vi "FRF_Koherenz_THD_Single_Shot.vi"(6 "error in":errorcluster, 7 "Peiker_Stepped Sweep Settings":T1={"Input Settings"={"IEPE min time to settle [s]"=0.0, "Responce Channel Settings"={"DSA response channel settings"={"coupling"=10045, "enable IEPE excitation"=FALSE, "IEPE current [mA]"=4.0}, "response channel info"={"sensor sensitivity"=200.0, "engineering units"=2, "dB reference"=2e-05, "custom label"="EU", "weighting filter"=0, "pregain"=0.0}, "AI response settings"={"response channel"="SOUNDACQ/ai1", "max value [V]"=10.0, "min value [V]"=-10.0, "terminal configuration"=-1}}, "Stimulus Channel Settings"={"AI stimulus settings"={"stimulus channel"="SOUNDACQ/ai0", "max value [V]"=10.0, "min value [V]"=-10.0, "terminal configuration"=-1}, "DSA stimulus channel settings"={"coupling"=10045, "enable IEPE excitation"=TRUE, "IEPE current [mA]"=4.0}, "stimulus channel info"={"sensor sensitivity"=11.4, "engineering units"=2, "dB reference"=2e-05, "custom label"="EU", "weighting filter"=0, "pregain"=0.0}}}, "Output Settings"={"AO source settings"={"excitation channel"="SOUNDACQ/ao0", "max value [V]"=10.0, "min value [V]"=-10.0, "terminal configuration"=-1}}} {"Output Settings"."AO source settings"."terminal configuration" items=["Default"=-1, "RSE"=10083, "Differential"=10106, "Pseudodifferential"=12529]; "Output Settings"."AO source settings"."min value [V]" format="%0.2f"; "Output Settings"."AO source settings"."max value [V]" format="%0.2f"; "Input Settings"."Stimulus Channel Settings"."stimulus channel info"."pregain" format="%.2f"; "Input Settings"."Stimulus Channel Settings"."stimulus channel info"."weighting filter" items=["Linear", "A-weighting", "B-weighting", "C-weighting", "ITU-R 468-4", "Dolby", "CCITT", "C-message", "Wb", "Wc", "Wd", "We", "Wf", "Wh", "Wj", "Wk", "Wm", "AES17 20 kHz lowpass", "AES17 40 kHz lowpass", "AES17 20 kHz highpass", "AES17 40 kHz highpass"]; "Input Settings"."Stimulus Channel Settings"."stimulus channel info"."dB reference" format="%^.1e"; "Input Settings"."Stimulus Channel Settings"."stimulus channel info"."engineering units" items=["custom..."=0, "V"=1, "A"=21, "C"=30, "pC"=31, "s"=32, "-"=29, "Pa"=2, "N"=20, "g"=3, "m/s^2"=4, "m/s"=5, "m"=6, "mm/s"=12, "mm"=13, "micron/s"=14, "micron"=15, "in/s^2"=7, "in/s"=8, "in"=9, "mil/s"=10, "mil"=11, "rad/s^2"=16, "rad/s"=17, "rad"=18, "deg/s^2"=26, "deg/s"=27, "deg"=28, "RPM"=22, "cycle/s^2"=23, "Hz"=24, "cycle"=25, "strain"=19]; "Input Settings"."Stimulus Channel Settings"."stimulus channel info"."sensor sensitivity" format="%#_5f"; "Input Settings"."Stimulus Channel Settings"."DSA stimulus channel settings"."IEPE current [mA]" format="%.1f"; "Input Settings"."Stimulus Channel Settings"."DSA stimulus channel settings"."coupling" items=["AC"=10045, "DC"=10050, "GND"=10066]; "Input Settings"."Stimulus Channel Settings"."AI stimulus settings"."terminal configuration" items=["Default"=-1, "RSE"=10083, "NRSE"=10078, "Differential"=10106, "Pseudodifferential"=12529]; "Input Settings"."Stimulus Channel Settings"."AI stimulus settings"."min value [V]" format="%.2f"; "Input Settings"."Stimulus Channel Settings"."AI stimulus settings"."max value [V]" format="%.2f"; "Input Settings"."Responce Channel Settings"."AI response settings"."terminal configuration" items=["Default"=-1, "RSE"=10083, "NRSE"=10078, "Differential"=10106, "Pseudodifferential"=12529]; "Input Settings"."Responce Channel Settings"."AI response settings"."min value [V]" format="%.2f"; "Input Settings"."Responce Channel Settings"."AI response settings"."max value [V]" format="%.2f"; "Input Settings"."Responce Channel Settings"."response channel info"."pregain" format="%.2f"; "Input Settings"."Responce Channel Settings"."response channel info"."weighting filter" items=["Linear", "A-weighting", "B-weighting", "C-weighting", "ITU-R 468-4", "Dolby", "CCITT", "C-message", "Wb", "Wc", "Wd", "We", "Wf", "Wh", "Wj", "Wk", "Wm", "AES17 20 kHz lowpass", "AES17 40 kHz lowpass", "AES17 20 kHz highpass", "AES17 40 kHz highpass"]; "Input Settings"."Responce Channel Settings"."response channel info"."dB reference" format="%^.1e"; "Input Settings"."Responce Channel Settings"."response channel info"."engineering units" items=["custom..."=0, "V"=1, "A"=21, "C"=30, "pC"=31, "s"=32, "-"=29, "Pa"=2, "N"=20, "g"=3, "m/s^2"=4, "m/s"=5, "m"=6, "mm/s"=12, "mm"=13, "micron/s"=14, "micron"=15, "in/s^2"=7, "in/s"=8, "in"=9, "mil/s"=10, "mil"=11, "rad/s^2"=16, "rad/s"=17, "rad"=18, "deg/s^2"=26, "deg/s"=27, "deg"=28, "RPM"=22, "cycle/s^2"=23, "Hz"=24, "cycle"=25, "strain"=19]; "Input Settings"."Responce Channel Settings"."response channel info"."sensor sensitivity" format="%#_5f"; "Input Settings"."Responce Channel Settings"."DSA response channel settings"."IEPE current [mA]" format="%.1f"; "Input Settings"."Responce Channel Settings"."DSA response channel settings"."coupling" items=["AC"=10045, "DC"=10050, "GND"=10066]; "Input Settings"."IEPE min time to settle [s]" format="%.1f"}, 8 "timeout(s)":dbl=10.0, 9 "Std_Deviation_Thresold":dbl=0.04, 10 "Excitation_amplitude(Vpeak)":dbl=0.35 min=0.0 format="%.3f", 11 "dB SPL":dbl=94.0502) -> (0 "mean":dbl=0.5389452537133329, 3 "Sensitivity(mVeff/Pa)":dbl=314.40385852797573, 4 "error out":errorcluster)   [LabVIEW 2018]
uses:
  <vilib>/addons/_NISVFA/_Shared subVIs/Controls/svc_Window [Dual FFT].ctl
  Peiker_Stepped Sweep Settings.ctl
  <vilib>/addons/_NISVFA/_Shared subVIs/Controls/svc_DSA Channel Settings.ctl
  <vilib>/addons/_NISVFA/_Shared subVIs/Controls/svc_Channel Info.ctl
  <vilib>/addons/_NISVFA/_Shared subVIs/Controls/svc_Engineering Units Text Ring.ctl
  <vilib>/addons/_NISVFA/_Shared subVIs/Controls/svc_Weighting Filter Text Ring.ctl
  <vilib>/DAQmx/write.llb/DAQmx Write (Analog 1D DBL 1Chan NSamp).vi
  <vilib>/DAQmx/read.llb/DAQmx Read (Analog 1D Wfm NChan NSamp).vi
  THD_Mess_Status.vi
  <vilib>/DAQmx/create/channels.llb/DAQmx Create Channel (AI-Voltage-Basic).vi
  <vilib>/DAQmx/configure/timing.llb/DAQmx Timing (Sample Clock).vi
  <vilib>/DAQmx/create/channels.llb/DAQmx Create Channel (AO-Voltage-Basic).vi
  <vilib>/DAQmx/configure/trigger.llb/DAQmx Start Trigger (Digital Edge).vi
  <vilib>/DAQmx/miscellaneous.llb/DAQmx Fill In Error Info.vi
  <vilib>/addons/_NISVFA/_Baseband FFT/SVFA Frequency Response (1x1) (Mag-Phase).vi
  <vilib>/addons/Sound and Vibration/svt_Distortion/SVT THD and Harmonic Components (Time) (1 Ch).vi
  <vilib>/addons/_NISVFA/_Baseband FFT/SVFA Power Spectrum (1 Ch).vi
  <vilib>/Analysis/NI_AALBase.lvlib
  <vilib>/addons/Sound and Vibration/svt_Distortion/SoundVib_Distortion.lvlib
  <resource>/objmgr/daqmx.rc
panel:
  out "Array 4":dbl[](array[numeric])
  out "Array 3":dbl[](array[numeric])
  out "Array 2":dbl[](array[numeric])
  out "standard deviation":dbl=0.020322606714807942
  out "Array":u32[](array[numeric])=[21, 20, 29, 17, 19, 19, 19, 19, 25, 19, 20, 18, 18, 22, 20, 18, 22, 19, 19, 23, 19, 19, 21, 20, 20, 19, 20, 19]
  out "XY Graph 3":cluster{dbl[], dbl[]}[](graph)=[{[0.021, 0.041, 0.07, 0.08700000000000001, 0.10600000000000001, 0.125, 0.144, 0.16299999999999998, 0.18799999999999997, 0.20699999999999996, 0.22699999999999995, 0.24499999999999994, 0.26299999999999996, 0.285, 0.305, 0.323, 0.34500000000000003, 0.36400000000000005, 0.38300000000000006, 0.4060000000000001, 0.4250000000000001, 0.4440000000000001, 0.46500000000000014, 0.48500000000000015, 0.5050000000000001, 0.5240000000000001, 0.5440000000000002, 0.5630000000000002], [0.5, 0.5, 0.5, 0.5, 0.5, 0.5, 0.5, 0.5, 0.5, 0.5, 0.5, 0.5, 0.5, 0.5, 0.5, 0.5, 0.5, 0.5, 0.5, 0.5, 0.5, 0.5, 0.5, 0.5, 0.5, 0.5, 0.5, 0.5389452537133329]}, {[0.021, 0.041, 0.07, 0.08700000000000001, 0.10600000000000001, 0.125, 0.144, 0.16299999999999998, 0.18799999999999997, 0.20699999999999996, 0.22699999999999995, 0.24499999999999994, 0.26299999999999996, 0.285, 0.305, 0.323, 0.34500000000000003, 0.36400000000000005, 0.38300000000000006, 0.4060000000000001, 0.4250000000000001, 0.4440000000000001, 0.46500000000000014, 0.48500000000000015, 0.5050000000000001, 0.5240000000000001, 0.5440000000000002, 0.5630000000000002], [0.5, 0.5, 0.5, 0.5, 0.5, 0.5, 0.5, 0.5, 0.5, 0.5, 0.5, 0.5, 0.5, 0.5, 0.5, 0.5, 0.5, 0.5, 0.5, 0.5, 0.5, 0.5, 0.5, 0.5, 0.5, 0.5, 0.5, 0.020322606714807942]}]
  in  "Coh Faktor Thresold":dbl=999.98 format="%#_10g"
  out "XY Graph 2":cluster{dbl[], dbl[]}(graph)={[0.021, 0.041, 0.07, 0.08700000000000001, 0.10600000000000001, 0.125, 0.144, 0.16299999999999998, 0.18799999999999997, 0.20699999999999996, 0.22699999999999995, 0.24499999999999994, 0.26299999999999996, 0.285, 0.305, 0.323, 0.34500000000000003, 0.36400000000000005, 0.38300000000000006, 0.4060000000000001, 0.4250000000000001, 0.4440000000000001, 0.46500000000000014, 0.48500000000000015, 0.5050000000000001, 0.5240000000000001, 0.5440000000000002, 0.5630000000000002], [0.0, 0.0, 0.0, 0.0, 0.0, 0.0, 0.0, 0.0, 0.0, 0.0, 0.545398761909948, 0.5338370932650872, 0.551146395387674, 0.5719764653070627, 0.5375454545895423, 0.537446460172108, 0.5808316642168437, 0.5322047145448163, 0.542195941406813, 0.5587662684664381, 0.535636496263525, 0.5091814361274755, 0.530595639527823, 0.5291564969244456, 0.5460569136668927, 0.5432199651402557, 0.5429647634305357, 0.513659110796227]}
  out "Big Sound Disturbances detected":i32=1
  out "Sound Pressure (Pa)":dbl=1.0081844522429841
  in  "swept sine settings":enum32{"DAQ Settings", "FRF Settings"}(tab)=enum."FRF Settings"
  out "input channel (response)":tag="SOUNDACQ/ai1"
  in  "propagation delay [samples]":i32=133 min=1 step=1
  out "input channel (stimulus)":tag="SOUNDACQ/ai0"
  out "output physical channel":tag="SOUNDACQ/ao0"
  out "actual update rate":dbl=50000.00001018634 format="%.2f"
  in  "sampling rate [Hz]":dbl=50000.0 format="%.2f"
  out "averages completed":dbl=5665.0
  in  "restart averaging":bool
  in  "averaging parameters":T6={"averaging mode"=enum."RMS averaging", "weighting mode"=enum."Exponential", "number of averages"=2, "linear mode"=enum."One shot"} {"number of averages" min=1 step=1}
  in  "view":T7={"dB On"=TRUE, "unwrap phase"=FALSE, "convert to degree"=TRUE}
  in  "block size":i32=1000 min=128
  in  "window":T8=1 items=["None"=0, "Hanning"=1, "Hamming"=2, "Blackman-Harris"=3, "Exact Blackman"=4, "Blackman"=5, "Flat Top"=6, "4 Term B-Harris "=7, "7 Term B-Harris"=8, "Low Sidelobe"=9, "Force - Exponential"=10, "Blackman Nuttall"=11, "Triangle"=30, "Bartlett-Hanning"=31, "Bohman"=32, "Parzen"=33, "Welch"=34, "Kaiser"=60, "Dolph-Chebyshev"=61, "Gaussian"=62]
  in  "Tab Control":enum32{"Getting Started", "Time Record", "FRF"}(tab)=enum."FRF"
  in  "Getting Started Text":string="GETTING STARTED\n\nThis VI measures the Frequency Response Function (FRF) of a device under test (DUT).  It generates a broadband stimulus signal to excite the DUT.  The magnitude and phase of the DUT output are compared to the stimulus signal to calculate the FRF.  \n\nRefer to the wiring diagram to physically connect the DSA or DAQ device to the DUT.  This example uses two analog input channels and one analog output channel.  Note that the analog output is connected to both the DUT input and to the first analog input channel on the measurement device.  \n\nThe wiring diagram assumes that you use the default channel settings.  If you change the channel settings in the VI front panel you should adjust the physical connections appropriately.\n\nNI strongly recommends that you take precautions to limit the effects of out-of-band aliasing in your frequency domain measurements.  DSA devices use transparent digital and analog hardware filtering to eliminate aliased input and output frequencies.  Multifunction DAQ devices are more susceptible to the effects of aliased frequencies.  If you are using a non-DSA measurement device, we recommend addressing potential aliasing through high sampling rates, built-in analog filters on S Series devices, and/or external analog filters.\n\n\nKEY PARAMETERS\n\nDAQ Configuration:  device propagation delay [samples]\n\nThis parameter quantifies the time, measured in sample intervals, between when a sample of data is generated on analog output and when it is read on the analog input.  Common sources of delay are analog or digital filters and propagation time for acoustical or mechanical signals.  The combined delay of the digital anti-aliasing and anti-imaging filters on the NI PCI-4451 and PCI-4551 devices is approximately 77 samples.  When using a multifunction E Series or S Series device, we recommend entering a delay of 1 sample.  An easy way to determine this delay for any given measurement system is to run SVT Measure Propagation Delay.vi.  This VI is available from the LabVIEW Functions palette under Sound and Vibration >> Calibration.\n\n\nSource Settings:  signal type\n\nThis control allows you to specify the type of stimulus signal you would like to generate.  All of the available signal sources are broadband stimuli with frequency content ranging from just above DC to the value specified in the \"Maximum Frequency of Interest\" control.  Note that if you use the \"Chirp\" or \"Frequency flat chirp\" signal types, you should select \"None\" for the window type.\n\nSource Settings:  maximum frequency of interest [Hz]\n\nThis setting controls the sampling rate for input and output.  The sampling rate is 2.5 times the value of this control.  Reducing the maximum frequency of interest may help if you encounter issues of data transfer bandwidth.\n\nMeasurement Settings:  frequency resolution [Hz]\n\nThis setting controls the width of a single frequency bin in the frequency response measurement.  Improving the frequency resolution requires more data points per average. Thus, the acquisition block size increases with finer frequency resolutions.  Improving (i.e. reducing) the frequency resolution may help if you encounter issues of data transfer bandwidth. \n\nMeasurement Settings:  window\n\nThis setting controls the time-domain window applied to the input signals before the frequency response function is calculated.  If you use the \"Chirp\" or \"Frequency flat chirp\" excitation types, you should not apply a window.\n\n\nMeasurement Settings:  settle time [s]\n\nThis control allows you to specify a time interval between when the stimulus generation starts and when the measurement actually begins. This time interval will be coerced to an integer number of data blocks.  If your DUT has a significant transient response to the start of a stimulus signal, select the appropriate settle time to allow this transient response to pass.\n"
  out "time record 2":waveform(dbl)[](graph)=[{"t0"=timestamp(3568218948.523604 s since 1904-01-01), "dt"=1.9999999995925458e-05, "Y"=array[1000 elements], "attributes"=variant("NI_ChannelName"=variant(string "stimulus"), "NI_UnitDescription"=variant(string "Volts"))}, {"t0"=timestamp(3568218948.523604 s since 1904-01-01), "dt"=1.9999999995925458e-05, "Y"=array[1000 elements], "attributes"=variant("NI_ChannelName"=variant(string "response"), "NI_UnitDescription"=variant(string "Volts"))}]
  out "Waveform Graph":dbl[](graph)=[0.0, 0.04386663174750649, 0.08704146050769919, 0.1288435934396373, 0.16861378593560036, 0.20572483830236563, 0.23959148707504105, 0.26967963497152625, 0.2955147739257053, 0.31668946836310685, 0.33286978070330375, 0.34380053775504105, 0.349309354949895, 0.349309354949895, 0.343800537755041, 0.3328697807033037, 0.3166894683631068, 0.2955147739257052, 0.2696796349715262, 0.23959148707504094, 0.20572483830236554, 0.16861378593560022, 0.12884359343963722, 0.08704146050769904, 0.04386663174750641, -1.4434796673928885e-16, -0.043866631747506574, -0.08704146050769931, -0.1288435934396374, -0.16861378593560047, -0.20572483830236568, -0.23959148707504113, -0.2696796349715263, -0.29551477392570535, -0.3166894683631069, -0.3328697807033038, -0.3438005377550411, -0.34930935494989507, -0.34930935494989507, -0.343800537755041, -0.33286978070330375, -0.31668946836310674, -0.29551477392570524, -0.2696796349715261, -0.23959148707504097, -0.2057248383023654, -0.16861378593560022, -0.12884359343963706, -0.08704146050769901, -0.04386663174750623, 1.9968971138109581e-16, 0.043866631747506754, 0.0870414605076994, 0.12884359343963755, 0.16861378593560059, 0.20572483830236585, 0.23959148707504127, 0.2696796349715264, 0.29551477392570547, 0.31668946836310696, 0.3328697807033039, 0.3438005377550411, 0.3493093549498952, 0.349309354949895, 0.3438005377550411, 0.33286978070330364, 0.3166894683631068, 0.2955147739257051, 0.2696796349715261, 0.23959148707504077, 0.20572483830236538, 0.16861378593560003, 0.128843593439637, 0.08704146050769881, 0.04386663174750615, -3.7825103292588036e-16, -0.04386663174750685, -0.08704146050769955, -0.12884359343963767, -0.1686137859356007, -0.20572483830236596, -0.23959148707504133, -0.2696796349715265, -0.29551477392570547, -0.3166894683631071, -0.33286978070330386, -0.3438005377550412, -0.34930935494989507, -0.3493093549498951, -0.34380053775504094, -0.3328697807033037, -0.31668946836310663, -0.29551477392570513, -0.2696796349715259, -0.23959148707504077, -0.2057248383023652, -0.1686137859356, -0.12884359343963683, -0.08704146050769876, -0.043866631747506, 4.652785860585762e-16, 0.043866631747506976, 0.08704146050769966, 0.12884359343963775, 0.1686137859356008, 0.20572483830236601, 0.23959148707504146, 0.2696796349715266, 0.29551477392570563, 0.3166894683631071, 0.33286978070330403, 0.34380053775504116, 0.3493093549498952, 0.349309354949895, 0.34380053775504105, 0.3328697807033036, 0.3166894683631067, 0.29551477392570497, 0.26967963497152597, 0.2395914870750406, 0.2057248383023652, 0.1686137859355998, 0.1288435934396368, 0.08704146050769856, 0.043866631747505935, -6.422136043446325e-16, -0.04386663174750707, -0.08704146050769981, -0.12884359343963786, -0.16861378593560095, -0.20572483830236613, -0.23959148707504155, -0.2696796349715267, -0.2955147739257057, -0.3166894683631072, -0.33286978070330403, -0.34380053775504127, -0.3493093549498951, -0.3493093549498951, -0.34380053775504094, -0.33286978070330364, -0.3166894683631066, -0.295514773925705, -0.2696796349715258, -0.23959148707504063, -0.20572483830236502, -0.1686137859355998, -0.12884359343963658, -0.08704146050769855, -0.04386663174750571, 6.790900307362957e-16, 0.04386663174750728, 0.08704146050769987, 0.12884359343963805, 0.168613785935601, 0.2057248383023663, 0.2395914870750416, 0.2696796349715268, 0.29551477392570574, 0.31668946836310724, 0.3328697807033041, 0.34380053775504127, 0.34930935494989523, 0.34930935494989507, 0.34380053775504105, 0.33286978070330353, 0.31668946836310663, 0.29551477392570485, 0.26967963497152586, 0.23959148707504044, 0.20572483830236507, 0.16861378593559959, 0.1288435934396366, 0.08704146050769831, 0.04386663174750571, -9.118275795874653e-16, -0.04386663174750731, -0.08704146050770008, -0.1288435934396381, -0.1686137859356012, -0.20572483830236638, -0.23959148707504177, -0.2696796349715269, -0.29551477392570585, -0.31668946836310735, -0.33286978070330414, -0.3438005377550414, -0.3493093549498952, -0.3493093549498952, -0.34380053775504094, -0.33286978070330364, -0.31668946836310646, -0.29551477392570497, -0.26967963497152564, -0.23959148707504052, -0.20572483830236482, -0.16861378593559964, -0.12884359343963636, -0.08704146050769833, -0.04386663174750547, 9.369539649348169e-16, 0.04386663174750753, 0.08704146050770015, 0.1288435934396383, 0.16861378593560128, 0.20572483830236651, 0.23959148707504188, 0.26967963497152697, 0.29551477392570596, 0.31668946836310735, 0.33286978070330425, 0.3438005377550413, 0.3493093549498953, 0.34930935494989507, 0.34380053775504105, 0.3328697807033035, 0.3166894683631066, 0.29551477392570474, 0.26967963497152575, 0.23959148707504027, 0.2057248383023649, 0.1686137859355994, 0.12884359343963642, 0.08704146050769809, 0.04386663174750549, -1.1476483283666405e-15, -0.043866631747507545, -0.08704146050770031, -0.12884359343963833, -0.1686137859356014, -0.20572483830236657, -0.23959148707504194, -0.2696796349715271, -0.29551477392570596, -0.3166894683631075, -0.3328697807033042, -0.3438005377550415, -0.3493093549498952, -0.34930935494989523, -0.3438005377550409, -0.33286978070330364, -0.3166894683631064, -0.29551477392570485, -0.26967963497152553, -0.23959148707504035, -0.20572483830236465, -0.16861378593559945, -0.12884359343963617, -0.0870414605076981, -0.04386663174750526, 1.1742316103832695e-15, 0.04386663174750774, 0.08704146050770038, 0.1288435934396385, 0.1686137859356015, 0.20572483830236668, 0.23959148707504208, 0.26967963497152714, 0.29551477392570613, 0.31668946836310746, 0.33286978070330436, 0.3438005377550414, 0.34930935494989535, 0.34930935494989507, 0.34380053775504105, 0.3328697807033034, 0.3166894683631065, 0.29551477392570463, 0.26967963497152564, 0.2395914870750401, 0.20572483830236474, 0.1686137859355992, 0.12884359343963622, 0.08704146050769787, 0.04386663174750527, -1.3799860776667061e-15, -0.04386663174750778, -0.08704146050770055, -0.12884359343963858, -0.1686137859356016, -0.2057248383023668, -0.23959148707504213, -0.26967963497152725, -0.29551477392570613, -0.31668946836310763, -0.3328697807033043, -0.34380053775504155, -0.34930935494989523, -0.34930935494989523, -0.3438005377550409, -0.3328697807033036, -0.3166894683631063, -0.2955147739257048, -0.26967963497152536, -0.23959148707504024, -0.20572483830236446, -0.16861378593559928, -0.12884359343963595, -0.08704146050769791, -0.04386663174750502, 1.3828050033151684e-15, 0.04386663174750799, 0.08704146050770059, 0.12884359343963872, 0.1686137859356017, 0.20572483830236687, 0.23959148707504224, 0.2696796349715273, 0.29551477392570624, 0.31668946836310763, 0.3328697807033044, 0.3438005377550415, 0.3493093549498954, 0.3493093549498951, 0.34380053775504105, 0.3328697807033034, 0.31668946836310646, 0.2955147739257046, 0.26967963497152553, 0.23959148707504, 0.2057248383023646, 0.16861378593559903, 0.12884359343963606, 0.08704146050769766, 0.04386663174750509, -1.6200419911821529e-15, -0.04386663174750797, -0.0870414605077008, -0.12884359343963875, -0.16861378593560186, -0.20572483830236696, -0.23959148707504235, -0.2696796349715274, -0.2955147739257063, -0.31668946836310774, -0.3328697807033044, -0.3438005377550416, -0.34930935494989535, -0.34930935494989523, -0.34380053775504094, -0.33286978070330353, -0.3166894683631063, -0.2955147739257047, -0.2696796349715253, -0.2395914870750401, -0.20572483830236435, -0.16861378593559911, -0.12884359343963578, -0.08704146050769773, -0.04386663174750482, 1.5683323238181723e-15, 0.04386663174750821, 0.08704146050770077, 0.12884359343963897, 0.16861378593560186, 0.20572483830236712, 0.23959148707504238, 0.2696796349715275, 0.29551477392570635, 0.3166894683631078, 0.3328697807033045, 0.3438005377550416, 0.3493093549498954, 0.3493093549498952, 0.343800537755041, 0.3328697807033034, 0.31668946836310635, 0.2955147739257045, 0.26967963497152536, 0.23959148707503988, 0.2057248383023644, 0.16861378593559886, 0.12884359343963583, 0.08704146050769745, 0.04386663174750486, -1.851539483798542e-15, -0.043866631747508184, -0.08704146050770104, -0.12884359343963894, -0.1686137859356021, -0.2057248383023671, -0.23959148707504258, -0.26967963497152747, -0.2955147739257065, -0.31668946836310774, -0.3328697807033046, -0.34380053775504155, -0.3493093549498954, -0.3493093549498951, -0.34380053775504094, -0.3328697807033034, -0.31668946836310624, -0.2955147739257045, -0.2696796349715252, -0.2395914870750399, -0.20572483830236418, -0.16861378593559892, -0.12884359343963558, -0.08704146050769754, -0.04386663174750459, 1.7499632927638065e-15, 0.04386663174750846, 0.08704146050770092, 0.12884359343963922, 0.16861378593560197, 0.20572483830236735, 0.23959148707504244, 0.2696796349715277, 0.29551477392570635, 0.3166894683631079, 0.3328697807033045, 0.34380053775504166, 0.34930935494989535, 0.3493093549498952, 0.3438005377550409, 0.33286978070330336, 0.31668946836310624, 0.2955147739257044, 0.26967963497152525, 0.23959148707503974, 0.20572483830236427, 0.1686137859355987, 0.1288435934396357, 0.08704146050769727, 0.04386663174750472, -2.041200325084147e-15, -0.043866631747508315, -0.08704146050770123, -0.12884359343963905, -0.16861378593560228, -0.2057248383023672, -0.23959148707504271, -0.2696796349715276, -0.29551477392570663, -0.31668946836310785, -0.33286978070330464, -0.3438005377550416, -0.34930935494989546, -0.3493093549498951, -0.34380053775504094, -0.33286978070330336, -0.3166894683631062, -0.2955147739257044, -0.2696796349715251, -0.23959148707503977, -0.20572483830236402, -0.16861378593559875, -0.1288435934396354, -0.08704146050769736, -0.04386663174750438, 1.9355244945847005e-15, 0.04386663174750867, 0.0870414605077011, 0.12884359343963941, 0.16861378593560214, 0.20572483830236754, 0.23959148707504258, 0.26967963497152786, 0.29551477392570646, 0.316689468363108, 0.33286978070330453, 0.3438005377550417, 0.34930935494989535, 0.3493093549498952, 0.3438005377550408, 0.3328697807033033, 0.31668946836310613, 0.2955147739257043, 0.2696796349715251, 0.23959148707503958, 0.20572483830236407, 0.1686137859355985, 0.12884359343963547, 0.08704146050769705, 0.0438666317475045, -2.2727655803363167e-15, -0.043866631747508524, -0.08704146050770145, -0.12884359343963925, -0.16861378593560247, -0.20572483830236735, -0.23959148707504288, -0.26967963497152764, -0.29551477392570674, -0.31668946836310785, -0.33286978070330475, -0.3438005377550416, -0.3493093549498955, -0.34930935494989507, -0.34380053775504094, -0.33286978070330325, -0.31668946836310613, -0.2955147739257043, -0.269679634971525, -0.23959148707503963, -0.20572483830236388, -0.1686137859355986, -0.1288435934396352, -0.08704146050769718, -0.04386663174750416, 2.119012159750716e-15, 0.043866631747508905, 0.08704146050770128, 0.12884359343963964, 0.1686137859356023, 0.20572483830236774, 0.23959148707504271, 0.269679634971528, 0.2955147739257066, 0.3166894683631082, 0.3328697807033046, 0.3438005377550418, 0.34930935494989535, 0.34930935494989523, 0.34380053775504077, 0.3328697807033033, 0.316689468363106, 0.29551477392570424, 0.2696796349715249, 0.23959148707503947, 0.20572483830236388, 0.16861378593559834, 0.12884359343963528, 0.08704146050769684, 0.043866631747504305, -2.5055505630325325e-15, -0.04386663174750871, -0.0870414605077017, -0.12884359343963941, -0.16861378593560272, -0.20572483830236749, -0.23959148707504313, -0.26967963497152775, -0.29551477392570696, -0.3166894683631079, -0.3328697807033049, -0.3438005377550416, -0.3493093549498956, -0.34930935494989507, -0.34380053775504094, -0.3328697807033032, -0.3166894683631061, -0.2955147739257042, -0.26967963497152486, -0.23959148707503947, -0.20572483830236368, -0.1686137859355984, -0.12884359343963497, -0.08704146050769695, -0.0438666317475039, 2.343509772090996e-15, 0.043866631747509176, 0.08704146050770149, 0.12884359343963991, 0.1686137859356025, 0.20572483830236798, 0.23959148707504288, 0.26967963497152825, 0.2955147739257067, 0.31668946836310835, 0.33286978070330464, 0.34380053775504194, 0.34930935494989535, 0.3493093549498953, 0.3438005377550407, 0.3328697807033033, 0.3166894683631059, 0.2955147739257042, 0.26967963497152475, 0.23959148707503936, 0.20572483830236368, 0.16861378593559817, 0.12884359343963506, 0.08704146050769664, 0.04386663174750407, -2.7489946083369965e-15, -0.04386663174750894, -0.08704146050770196, -0.1288435934396396, -0.168613785935603, -0.20572483830236765, -0.23959148707504338, -0.2696796349715279, -0.2955147739257072, -0.316689468363108, -0.3328697807033051, -0.34380053775504166, -0.34930935494989573, -0.349309354949895, -0.343800537755041, -0.3328697807033031, -0.3166894683631061, -0.295514773925704, -0.2696796349715248, -0.23959148707503927, -0.20572483830236357, -0.16861378593559817, -0.1288435934396348, -0.08704146050769672, -0.043866631747503694, 2.579533808777512e-15, 0.04386663174750942, 0.08704146050770172, 0.12884359343964016, 0.1686137859356027, 0.20572483830236823, 0.23959148707504305, 0.26967963497152847, 0.2955147739257068, 0.3166894683631085, 0.3328697807033047, 0.34380053775504205, 0.34930935494989535, 0.34930935494989535, 0.34380053775504066, 0.3328697807033033, 0.3166894683631058, 0.29551477392570413, 0.2696796349715246, 0.23959148707503924, 0.20572483830236346, 0.168613785935598, 0.1288435934396348, 0.08704146050769644, 0.043866631747503805, -2.9610781058023172e-15, -0.0438666317475092, -0.08704146050770217, -0.12884359343963986, -0.1686137859356032, -0.20572483830236787, -0.23959148707504355, -0.2696796349715281, -0.2955147739257073, -0.31668946836310813, -0.33286978070330514, -0.34380053775504166, -0.34930935494989573, -0.34930935494989496, -0.343800537755041, -0.332869780703303, -0.316689468363106, -0.29551477392570386, -0.2696796349715247, -0.23959148707503905, -0.20572483830236343, -0.16861378593559792, -0.12884359343963464, -0.08704146050769646, -0.043866631747503514, 2.844641568740952e-15, 0.0438666317475096, 0.08704146050770196, 0.12884359343964033, 0.16861378593560292, 0.2057248383023684, 0.2395914870750432, 0.2696796349715286, 0.2955147739257069, 0.31668946836310863, 0.33286978070330475, 0.34380053775504216, 0.34930935494989535, 0.3493093549498954, 0.3438005377550406, 0.3328697807033033, 0.3166894683631057, 0.2955147739257041, 0.2696796349715244, 0.23959148707503913, 0.20572483830236324, 0.16861378593559787, 0.12884359343963456, 0.08704146050769626, 0.04386663174750354, -3.166886783194378e-15, -0.04386663174750946, -0.0870414605077024, -0.1288435934396401, -0.16861378593560342, -0.20572483830236807, -0.23959148707504377, -0.2696796349715282, -0.29551477392570746, -0.3166894683631082, -0.33286978070330525, -0.34380053775504166, -0.3493093549498958, -0.3493093549498949, -0.343800537755041, -0.33286978070330286, -0.31668946836310596, -0.2955147739257037, -0.2696796349715246, -0.23959148707503886, -0.2057248383023633, -0.1686137859355977, -0.12884359343963447, -0.08704146050769622, -0.043866631747503326, 3.074919333913295e-15, 0.04386663174750979, 0.08704146050770217, 0.12884359343964052, 0.16861378593560308, 0.20572483830236857, 0.23959148707504332, 0.26967963497152875, 0.29551477392570696, 0.31668946836310874, 0.33286978070330475, 0.3438005377550422, 0.3493093549498953, 0.3493093549498954, 0.3438005377550405, 0.33286978070330325, 0.3166894683631055, 0.29551477392570397, 0.26967963497152425, 0.239591487075039, 0.20572483830236307, 0.1686137859355977, 0.12884359343963436, 0.08704146050769608, 0.04386663174750335, -3.353234031590324e-15, -0.04386663174750964, -0.08704146050770258, -0.12884359343964025, -0.16861378593560358, -0.20572483830236818, -0.2395914870750439, -0.2696796349715283, -0.2955147739257076, -0.31668946836310824, -0.33286978070330536, -0.34380053775504166, -0.34930935494989584, -0.34930935494989485, -0.343800537755041, -0.33286978070330275, -0.3166894683631059, -0.2955147739257035, -0.2696796349715245, -0.23959148707503866, -0.20572483830236313, -0.16861378593559748, -0.12884359343963425, -0.087041460507696, -0.04386663174750309, 3.2855662635000726e-15, 0.043866631747510036, 0.08704146050770237, 0.12884359343964077, 0.16861378593560325, 0.2057248383023688, 0.23959148707504346, 0.2696796349715289, 0.2955147739257071, 0.31668946836310885, 0.3328697807033048, 0.34380053775504227, 0.3493093549498953, 0.3493093549498954, 0.34380053775504044, 0.3328697807033032, 0.3166894683631054, 0.29551477392570386, 0.2696796349715241, 0.23959148707503883, 0.20572483830236285, 0.16861378593559748, 0.1288435934396341, 0.08704146050769583, 0.04386663174750308, -3.614242152089053e-15, -0.043866631747509904, -0.08704146050770284, -0.1288435934396405, -0.16861378593560383, -0.2057248383023684, -0.2395914870750441, -0.26967963497152847, -0.29551477392570774, -0.31668946836310835, -0.3328697807033055, -0.3438005377550417, -0.3493093549498959, -0.34930935494989485, -0.34380053775504094, -0.3328697807033027, -0.3166894683631058, -0.2955147739257034, -0.2696796349715243, -0.2395914870750385, -0.2057248383023629, -0.16861378593559728, -0.128843593439634, -0.08704146050769578, -0.04386663174750282, 3.528319129919577e-15, 0.04386663174751031, 0.08704146050770262, 0.12884359343964102, 0.16861378593560347, 0.205724838302369, 0.23959148707504366, 0.2696796349715291, 0.29551477392570724, 0.31668946836310896, 0.3328697807033049, 0.3438005377550423, 0.34930935494989535, 0.3493093549498954, 0.34380053775504044, 0.33286978070330314, 0.31668946836310535, 0.29551477392570374, 0.269679634971524, 0.23959148707503866, 0.20572483830236268, 0.16861378593559728, 0.12884359343963392, 0.08704146050769561, 0.04386663174750286, -3.8537966220997255e-15, -0.04386663174751014, -0.08704146050770308, -0.12884359343964075, -0.16861378593560405, -0.20572483830236862, -0.2395914870750443, -0.26967963497152864, -0.2955147739257079, -0.31668946836310846, -0.3328697807033056, -0.34380053775504177, -0.34930935494989596, -0.34930935494989485, -0.34380053775504094, -0.33286978070330264, -0.31668946836310574, -0.2955147739257033, -0.2696796349715242, -0.23959148707503833, -0.20572483830236277, -0.16861378593559706, -0.12884359343963384, -0.08704146050769553, -0.04386663174750262, 3.7827000646389886e-15, 0.04386663174751052, 0.08704146050770285, 0.12884359343964125, 0.1686137859356037, 0.20572483830236923, 0.23959148707504382, 0.2696796349715293, 0.29551477392570735, 0.31668946836310913, 0.332869780703305, 0.34380053775504243, 0.34930935494989535, 0.34930935494989546, 0.3438005377550404, 0.33286978070330314, 0.31668946836310524, 0.2955147739257037, 0.2696796349715238, 0.23959148707503855, 0.2057248383023625, 0.16861378593559712, 0.1288435934396337, 0.0870414605076954, 0.043866631747502625, -4.087089824564294e-15, -0.043866631747510376, -0.08704146050770332, -0.12884359343964097, -0.16861378593560428, -0.20572483830236882, -0.23959148707504452, -0.2696796349715288, -0.2955147739257081, -0.3166894683631086, -0.3328697807033057, -0.3438005377550418, -0.349309354949896, -0.34930935494989485, -0.34380053775504094, -0.3328697807033026, -0.3166894683631057, -0.2955147739257032, -0.2696796349715241, -0.23959148707503816, -0.2057248383023626, -0.16861378593559687, -0.12884359343963364, -0.0870414605076953, -0.0438666317475024, 4.020391062165701e-15, 0.043866631747510744, 0.08704146050770309, 0.12884359343964147, 0.16861378593560392, 0.20572483830236943, 0.23959148707504402, 0.26967963497152947, 0.2955147739257075, 0.3166894683631093, 0.3328697807033051, 0.34380053775504255, 0.3493093549498954, 0.3493093549498955, 0.3438005377550404, 0.33286978070330314, 0.3166894683631052, 0.29551477392570363, 0.2696796349715237, 0.23959148707503844, 0.20572483830236232, 0.16861378593559695, 0.12884359343963347, 0.08704146050769519, 0.04386663174750238, -4.3253296994408275e-15, -0.043866631747510626, -0.08704146050770357, -0.1288435934396412, -0.16861378593560453, -0.20572483830236904, -0.23959148707504474, -0.26967963497152897, -0.2955147739257083, -0.3166894683631087, -0.33286978070330586, -0.3438005377550419, -0.3493093549498961, -0.34930935494989485, -0.343800537755041, -0.33286978070330253, -0.3166894683631057, -0.2955147739257031, -0.26967963497152403, -0.239591487075038, -0.2057248383023625, -0.16861378593559667, -0.12884359343963347, -0.0870414605076951, -0.043866631747502195, 4.235794928784259e-15, 0.04386663174751099, 0.0870414605077033, 0.12884359343964172, 0.1686137859356041, 0.20572483830236968, 0.23959148707504418, 0.2696796349715297, 0.29551477392570763, 0.31668946836310946, 0.33286978070330514, 0.34380053775504266, 0.3493093549498954, 0.34930935494989557, 0.3438005377550403, 0.33286978070330314, 0.3166894683631051, 0.2955147739257036, 0.26967963497152353, 0.23959148707503833, 0.20572483830236213, 0.1686137859355968, 0.12884359343963325, 0.08704146050769501, 0.043866631747502154, -4.5256496033346805e-15, -0.04386663174751085, -0.08704146050770378, -0.1288435934396414, -0.16861378593560475, -0.2057248383023692, -0.23959148707504493, -0.2696796349715291, -0.29551477392570846, -0.31668946836310874, -0.332869780703306, -0.3438005377550419, -0.3493093549498962, -0.3493093549498948, -0.343800537755041, -0.3328697807033024, -0.31668946836310563, -0.2955147739257029, -0.2696796349715239, -0.2395914870750378, -0.20572483830236232, -0.16861378593559645, -0.12884359343963325, -0.08704146050769486, -0.04386663174750195]
  out "phase":cluster{"f0":dbl, "df":dbl, "magnitude":dbl[]}(graph)={"f0"=0.0, "df"=50.000000010186355, "magnitude"=[180.0, 134.27606914828107, 133.5615510807004, -80.26992245308311, -122.87427678007059, -95.82501017730308, -51.8601995664901, 151.69017113267955, -157.22561740749973, -59.866479908737055, -114.56789004679894, -151.29626637511112, -145.21845895760904, -101.88621488825433, 126.53430010424495, 120.26721751908497, 171.9100029832925, -163.74337093626585, -106.23143602227621, 6.13740887991103, 6.09478886540422, 6.060506613851925, -58.42051043475751, -24.72081136642481, -93.95757126204302, -177.22645941104443, 133.9534656366225, -161.16743351792613, -94.2469845422241, 7.8682815475159105, 102.83657397418624, -88.95619035046337, 64.31072185201634, 11.8946158990233, -48.58234755263293, 176.38948131746372, 61.91169670302172, -70.48817292654194, -53.0875437630805, -46.47863252755127, -26.354654620074385, -26.636760379066178, -74.35409468416377, -56.92429828365852, 18.466408402681278, -39.186887618054364, -26.822986479246072, -70.64947350846863, -24.122789691324915, 10.697713818408259, 3.7337339696406375, -6.213868474799509, 41.706081147063266, 117.87351463791273, 144.69248667673997, -149.32237283560974, -171.260788218224, 108.94694600216694, 110.83674649247514, 81.48989562812338, -40.44353698051692, -37.30772358674808, 49.97395696072729, 68.50324343584414, 102.70565945767542, 68.22720227220587, 38.32804609286374, -16.730418905408662, -85.97976201781469, 146.67308674611104, -161.9954529810673, -91.25318053201576, -88.73836695952998, 57.9523583234101, -1.166105125562501, -47.4475670882271, 111.10400573409613, -17.34908527602457, -84.40483992940568, -121.90697653667326, 9.64624489039396, -117.18080217401352, -168.51835221272722, 93.21736858716145, 132.24331110747312, 103.64723821859967, 71.71070955438955, 43.86332406301133, -158.01814776680447, -41.6202430838354, -73.77153382642871, -147.2588362537482, 175.84531695751897, 176.58267216672996, -42.59382988108921, 146.5898699151385, -174.9412893324381, 137.07571036664123, 50.35806834696832, -4.77684457187477, -79.33773381363126, -109.5363727629897, -160.62430515592135, -97.20042156113061, 150.68708356433294, 158.04791392375907, -153.81260206827898, 168.17535959640858, 171.14443780691877, 178.16961150172878, 130.72203240436588, 178.64528802192262, -144.06451903234128, 175.71422913288242, -128.4938664237058, -23.896715786933584, 41.152073755880814, 90.30054525841948, 23.80381586860164, -40.77768454999053, -77.78946642790513, -96.86632936331303, -39.36565051466159, -8.506531468579984, 13.545529882387415, -32.73050095169317, 52.84324048907252, 7.283476629283953, 51.22980209213097, 16.211913330384274, -114.64075379785685, 67.15240651557757, -172.5004686750056, -170.03794448460778, 88.2281480181498, 32.65913418398779, 176.02150850205902, 116.7548316620157, 125.54381294855169, 17.069184173969532, -8.727742639640974, -11.614469986293994, -8.415312798336359, 96.42446829935976, 94.97760083978626, 128.78565502421372, 111.41357148351018, 118.18311530159663, -54.40050115444829, -42.343109880882864, 15.190540530931251, -85.52854166153554, -87.3985513818599, -19.257422718167554, -11.660427557244954, -40.560921974648075, 63.63469835491003, -11.245643980320942, -104.88529024415953, 81.13884994293977, 144.75115920256576, 135.055475078031, 143.54177340267222, 82.79381894965331, -157.32247813655331, -117.96612109395865, -79.0200205887658, -77.55873373930896, -88.85265997350915, -137.71637896607405, -176.583461433106, -36.360702506419514, -39.93609976726301, -95.2659042520502, 104.83316573680995, 99.9561804609795, 11.498852589757485, 112.16724228767241, -52.387522613670875, -70.21116485581467, -68.45546036970272, 9.202861511608628, 113.30687127447125, 22.560658460580868, 128.58059948782736, 143.24437683504584, 138.19038129881238, 84.49803183732935, 99.35083169568179, 48.72150553018085, -11.239337099337456, 158.37882681768284, 149.07082734511067, -149.84751734971098, -62.86257052208094, 70.84026306218456, -160.25537258293414, 161.80326454611435, 87.40700105049594, 45.70570716921485, 177.76181776353778, -53.70863451120121, -22.994232001354312, 56.59949784662309, 85.2995314749204, 137.81340021050522, -135.66095519283257, -160.9210514873808, 143.51767458657667, -50.46886503401523, 68.57362950975708, 109.0223301324963, -86.54058432575577, -74.21713497902141, -46.165857656730715, 0.3689361403919183, 124.35509295852762, -179.2486463974101, -94.4824897705305, -54.91924002586894, -61.91999744833526, -82.7858531088168, -35.277591957168866, -78.4224096929908, -95.2914746895131, 81.35737785619358, -46.10569945407268, -108.70642903445066, -151.20823209329174, 30.59870611026655, -25.29063627998968, -15.670469000482104, 141.44093485396436, 67.98672822082946, 76.04721133261468, 63.74297939160055, -57.353402447894716, -128.0182627693445, 100.33506417823462, 100.37028488876679, 43.79348283227455, 4.24956029743411, 132.51731848481074, -168.90112169088377, -64.59875740083604, -106.6690611841177, 176.848396785602, -159.05167063027335, -139.44678777012012, -156.48290521450207, 81.4932328354058, 125.07575907626222, -84.92919930048804, -104.04321216004664, 137.8226871039259, 171.4668894711293, -133.69976674305573, -126.25569268186587, 141.68342354599605, 134.71323489308463, 156.52859257341117, -177.6121452098254, 119.25629376299818, 15.586535081854866, -59.09673936595464, -75.25450183816594, -71.93014065389382, 105.12037524265322, 79.42560347832477, -174.88471940979403, 153.15207042348706, 40.786546476525785, -22.981576946638874, 97.80443519168558, -128.09626285614146, -17.340433133834207, 65.57906753989296, 13.223919168669443, -130.90707920898942, 62.34622772246482, -3.512172450420756, 43.78191143291607, 80.970214212171, 92.43829845072923, 73.83517731042046, 99.27541896612159, -119.41326166864921, -25.06789064260184, 4.05855847569646, 166.74354359014495, 133.23980084475977, 43.11975038062648, -17.200073666149553, 143.63517217105735, 118.98661980533491, 46.84745068376606, 106.87655352650457, 152.34755263597125, 170.6673239228504, 85.53960808733311, 35.94158597158317, 32.23098223856609, -119.164333095034, -120.13560464880459, -34.8839868070259, -69.16400195868775, 48.81795423600886, 28.756355074747464, 160.81948254983, -152.24382375510402, 130.82192870600005, 156.68021467968927, -108.27876778977578, -50.71574578272773, -10.000794657507333, 40.73687893823096, -75.62620812968368, -84.72123512156759, 35.39997906503908, 166.4275633584039, -177.45442320593347, -56.56726075279851, -19.78635714575615, -22.803162173078974, 127.92473411992422, 18.225100734544746, -52.15392758233122, -55.76137274919576, -21.74282721425712, -55.38431553759938, -151.17098667419717, -27.60457005831463, -172.11618386029122, -170.21744870704293, -93.6481726257851, -6.288686706801815, -146.32587960753727, -26.715876114397943, -49.59037598461337, 39.0077710000312, 122.32714286596243, 37.898745711745875, 107.0548155903622, 167.11086653773458, 16.384059919615908, 25.251317759522497, 16.337397675226157, -70.65804932601722, -58.261782088015075, -35.72759658816851, 104.23364156917445, -28.892544454370796, -47.28854157771112, 54.28243704933181, 175.89688549455911, 111.14154816579651, 107.60923189622436, 55.33641477367048, -25.339077255017646, -98.90298017670813, -100.14853100075175, -14.689598571956484, 149.02245776685783, -175.86704204084666, -63.43234457090579, -126.33649487569771, -156.19898936193277, 169.20804510740965, -44.95779487637909, -122.09900510205767, -171.80637234104904, -22.05615873211294, -55.35160405044617, -171.62806036948913, 117.30328172271794, 73.93821296790885, 82.33531628675387, 128.3842932745579, 138.86825471611635, -70.27433453371742, -42.67177907153664, -7.413121873716856, 54.949397818001174, -139.31455367551087, -94.7356080198861, 166.1383022271507, 70.94066167595416, 82.15820143753639, 92.03919232482552, -77.51688133003765, -42.66659305184547, 6.919660334615624, -44.11046987229526, 25.95770179966253, 137.78930418300536, 157.62614009094236, 68.99379070000417, 93.53475980539127, 128.60881978239112, 36.02114768734927, -55.993392413823095, -82.23171240647775, -116.09456721194299, 91.51261496688018, 95.36331423372614, 149.11172203429055, 171.01737859783594, -160.91515968645376, 61.99934233352007, 54.93561576434196, 81.31074385278328, -175.1481932940273, 110.35378121191312, -78.5857243364054, -123.74480969967317, 72.1862788694128, 135.85489464537434, 113.36110375235698, 96.43867698123134, -9.737734095777034, -45.07693023511141, -46.26712604112423, 22.37846681417283, 9.543860473726898, -73.82271235101364, -151.0884390635147, 56.25525209312814, 93.52048005162325, 84.92651040283253, -49.31793282639124, -126.76669835351763, 160.7093688315058, 127.88673926399832, 98.46455389625599, 0.17312938166782862, 19.325872596446104, 97.63617953240198, -48.3609295551954, -100.77523963655892, -76.99005225408693, -41.23500652212819, -56.19026684637527, 12.364710378219112, 171.27080599107725, -119.65864033908306, -140.60786406215016, 175.17836362598092, -109.94274694742215, 21.93392345516276, -137.83949857189316, -130.98797719515403, -103.22083525329701, 171.96362896354262, 162.6369372946668, 164.16263694575065, 174.02473712524682, -95.21801528710907, -88.03581685335476, -115.03580560963962, -131.52812911703572, -35.99308300140727, 59.84996545393363, 11.845795305676532, 154.46227753677542, 154.7347711793267, 59.216672795959546, 70.00090365272072, -9.639442650017632, 88.56694758363923, 80.56946204333057, 37.78096801027596, 13.914667569190085, 8.13041473997635, -178.2678092229685, -168.02771888136473, 138.4515730100643, -11.472871266794266, -93.98668706172593, -159.1678023480476, 0.41817356061112176, 169.2326594683201, 171.64929120855098, 75.82821776334822, 25.987307144564156, -89.7722941073391, 125.15545365897603, 81.74470362105335, 34.799579893841354, 82.77528988536213, 54.508648107101855, 56.38321034318717, 39.83176085017427, 61.32858989774304, 11.3239241589915, -130.85540167760814, -135.260049812035, -173.0849376226668, 81.65890341799037, -19.59700579282434, -91.88333477801771]}
  out "mag":cluster{"f0":dbl, "df":dbl, "magnitude":dbl[]}(graph)={"f0"=0.0, "df"=50.000000010186355, "magnitude"=[30.32645571027238, 33.35016877260819, 51.65630582781234, 46.039555597294964, 42.228857804380915, 33.041716469511, 39.16622658643955, 37.106652476153904, 39.93356088413478, 24.787595039199203, 19.042376478795536, 28.2862292563792, 40.817782621382335, 33.08087955102327, 36.261520774346224, 36.10974970460068, 30.341249204871545, 28.439197363952008, 37.17242408901548, 2.1429045283726773, 2.1430531272694773, 2.1476981224947638, 38.318620771372224, 34.642555289442285, 43.23174614654822, 39.29061062951498, 40.117894692007965, 50.04210618789185, 44.03353706466616, 36.793225603410534, 21.397438358327534, 33.70510081833141, 41.08765844836383, 36.86431518306114, 33.55961022837638, 33.99524448568725, 29.823093556999886, 30.92223276317213, 25.41614639972267, 54.492772577378204, 61.82602513515203, 48.49456788351048, 31.34159554663727, 23.964448287231942, 23.892376729638386, 23.787608626535253, 28.429137085458468, 22.130621642839298, 17.274993404232667, 27.602526700529253, 30.715132248681943, 19.27548844323449, 26.110992609633126, 27.968850989221202, 18.76720441405345, 26.81797509848563, 32.376695284523564, 29.691762163716714, 25.03490148526971, 33.41424816275438, 42.43042924277563, 39.81365737900491, 19.47486938846334, 10.748931548877819, 26.139077970958887, 27.46277078217077, 26.196823336028686, 27.924336261602946, 21.262194227474865, 20.407866780953825, 16.17181475530155, 24.892273381208195, 21.068264165084145, 26.18063468910053, 26.1691980401407, 26.516793266047635, 20.46641151500392, 15.095692763069186, 25.80379238894915, 18.479364415940097, 30.424512942932346, 30.377634140594637, 27.830858990652892, 11.708498482973937, 24.9840508788095, 23.053111159994458, 19.904400410031965, 13.153279904973047, 24.150658573336226, 23.66162209516932, 9.172055890757175, 19.59967561562334, 21.37836084925256, 16.798690293855017, 22.58777775926528, 16.82083436894977, 25.58932958591285, 14.752505608341245, 15.69362314241356, 32.007175512605656, 31.664546175480467, 24.0286035694711, 22.650983860173135, 28.235332415535655, 19.57387916415157, 15.44158702976308, 26.474403039470438, 26.97834704800789, 28.1613921614923, 26.976679089535626, 25.849287121745633, 25.79037342094429, 12.653666890113124, 7.069365384266836, 18.055349997425775, 22.335943965142246, 24.813200741155292, 24.30423141865775, 14.484919290258976, 14.964289939486301, 24.984765831837258, 18.220791225885364, 21.163984636821567, 19.75424473940949, 18.78282227755991, 24.75129329619279, 11.382366765620402, 17.185609724393366, 13.387076215474798, 17.38577623098571, 7.853719487383252, -0.6214684261348745, 15.868294753461276, 26.044955969002924, 20.547185067083248, 19.824135422016877, 16.217575178258784, 17.193346001238893, 16.602284228421198, 16.537076506138245, 13.286457859996359, 13.911321859604822, 9.347328887077973, 13.667603430672639, 14.939426310389834, 11.371261515084544, 8.768616908205155, 18.334680332951027, 26.8433021051489, 24.908572008961315, 14.347785499780102, 21.876561478435782, 20.935297479723133, 19.624935938712756, 18.625123217735908, 19.279183842045992, 16.177385741442528, 7.050278492702251, 22.713294220928407, 11.911808070417887, 11.982620268154037, 15.330802435051282, 13.14787372927622, 2.491817830440267, 6.4223736072980735, 19.72843206823575, 19.54488647898829, 24.474887686197746, 20.874736815121633, 17.27396782338295, 6.912309883265756, 6.611313030746597, 16.5431681979964, 16.44703008634814, 15.855839823029235, 17.323478952795355, 20.313374045365613, 13.507650571425632, 14.161305670406414, 17.118253954627157, 14.65719440936348, 3.972565500616172, 8.512875634070475, 16.95836465347012, 21.35461507601576, 18.644628149884582, 21.087180844908673, 15.398667744532146, 18.468093480629413, 12.897465659932994, 21.230320987417457, 16.314919024747333, 12.397764662307754, 12.305731808489778, 22.446954785481516, 13.23733452092185, 11.511614077514347, 8.94980936927663, 18.06718794233462, 12.402353832152368, 7.79079318168666, 15.956192264161146, 6.050619678778878, 20.194057931230887, 18.54278998301126, 9.161229023568747, 8.244244470875532, 17.900071987778386, 18.59844261732054, 18.75843771967496, 19.801704283871583, 9.655899115636906, 13.570143586410719, 12.991903549366473, 15.92886730996515, 19.172575683650184, 13.817112405621065, 21.23005572060893, 3.9736687581379737, 14.669174834485474, 10.210344781268809, 9.571600093013693, 15.691959221828586, 21.617870817206224, 17.705625255527522, -3.60207877722432, 13.402518506471717, 20.912522118492994, 21.34303140295897, 15.214413174813185, 23.299538927389936, 16.532786082186313, 16.00452049462867, 6.513972531220978, 23.73981640477409, 15.493614633701338, 14.713075490604998, 8.256895275060671, 1.8180160838286887, 17.169491749255357, 16.591926907236306, 15.080957508650654, 13.140822157086474, 18.238029090478957, 15.065345898902772, 18.02619603556033, 16.834565216749866, 16.708144592906798, 15.482174885134546, 5.6077671485822105, 14.88523120935373, 7.702956645337183, 4.774241569332684, 6.4763451558267695, 9.37520263727002, 1.9068159773789206, 15.757020781474047, 19.315310735269826, 15.28775473144032, 3.068954159927968, -1.0618105791519659, 2.5335494776106775, 20.440839515885486, 18.52237973380394, 13.342526230776548, -3.0524827264182757, -2.507982711901027, 9.715826819363635, 5.59749900218522, 9.486483766550275, 13.523599098848592, 19.327613384482856, 13.986653840446335, 12.042488985595199, 15.12505687958798, 10.906618970542567, 17.46610754169853, 15.959172571732093, 17.827593836118453, 16.000990688239977, 15.67895681565987, 13.461983370887635, 19.59871608240568, 20.926159321002803, 16.404466448464262, 13.489808144097378, 11.353551705901449, 13.891820759777948, 11.489758123980566, 14.436807616091246, 11.919585915662518, 14.912417350868788, 14.791917437711655, 7.035768000001772, 9.219387965306522, 13.253272166062938, 5.318779879872509, 12.230807877296044, 9.583761479359643, 10.10129097378872, 10.780747124483984, -2.3736345415431868, 10.642655988478255, 16.962560779870234, 20.00003793907247, 17.89871694314852, 11.673603960940167, 16.532916709138437, 9.340935067679805, 12.28363524372215, 12.616557949777501, 21.004554835050676, 17.789771737117363, 12.844839581596045, 12.078645247870806, 8.213619041956248, 7.628471461001927, 9.845583507525946, 7.037523640662897, 12.457320364081522, 13.863426938670882, 4.924696309583833, 14.553542814272722, 20.029052064025517, 11.051914337300266, 13.853107735068807, 11.325094572283337, 11.0598116441162, 8.771575546104609, 10.867029035719334, 14.402237383757617, 2.8950907722126615, 13.103687690129142, 12.531465868517316, 10.872788847825998, 8.065027530199067, -4.590930822846304, 4.869639782995506, 8.378169860218303, 9.69763120384829, 5.728043000832784, 3.3426516483633923, 14.28646423954148, 7.567405819588133, 7.360454640341843, 11.076437778747227, 9.99295223279059, 8.432410709412196, 23.218990410529937, 16.931098452543644, 16.99886220166659, 16.067180221812517, 17.45474990743197, 11.296100174341339, 12.399112708565124, 9.237357861671713, 16.18176683973398, 14.714970718551239, 12.366436204502104, -2.6345827698629987, 3.6280477897275283, 2.418856085685805, 17.598665880832037, 18.18047053017954, 10.85034672638302, 14.180125077493269, 5.102370571628417, 12.427962021842207, 9.145012496578795, 17.23922844691504, 8.162111485043534, 4.225551779604247, 9.02090773758289, 15.811316999593995, 14.43475419678991, 12.94972934892809, 16.826771342917645, 8.745236019721682, 8.652224664955915, 3.3560665358198785, 13.86213200862059, 18.724012200586266, -12.368758934095453, 12.00831226575055, 9.826311948257553, 5.504354493547145, 15.714545433182279, 15.428780003307065, 9.100357704559203, 5.555947813599401, 3.7958455320155355, 8.36395597892444, 14.195169528000658, 6.358553231366653, 20.436261514300902, 19.265527975846993, 13.42976080842292, 12.311736587125194, 14.650228958121303, 10.301843242448882, 5.9243021557165125, 7.20868308546283, 6.976610038681735, 4.726036018000496, 10.124384242002538, 15.33781232952467, 15.007605083606135, 7.468312279583568, 7.1704661300228825, 11.508408889639377, 5.426869915293726, 8.797205624116577, -14.475476288516854, 18.119086302032805, 5.905907003244469, 13.510193811089719, 8.455881987026125, 13.605848114070188, 15.002017670923273, 4.8452117386542595, -2.8372984811800683, -0.4579066492094176, 5.270145843618945, 3.850208474989589, -10.901161302458025, 10.314470242833458, 8.579536211124974, 12.597971108447885, 9.460569852326548, 7.4156178278337475, 9.349774360209741, 11.442801538444119, 5.584129353370416, 11.504049065904915, 11.957345828273924, 5.358232176080461, -12.061347247426514, 9.407000053192222, 16.76481177385156, 11.712530628887798, 20.243074603077666, 16.76417456656016, 9.374216971458262, -5.942000942156861, 4.967476204058902, -0.2817732636847408, -0.058534793120438126, 6.116274229177976, 3.1789842844138954, -2.056708431934646, 15.177437823297486, 9.732841840424749, 7.254177538056329, 8.715871394220246, 14.280441176871912, 8.583185366106, 9.507660395482171, 16.21827808698299, 21.11756673935673, 6.675872146810164, -5.693065658514045, 1.4734738923862785, 11.48646664382536, 11.331469290605117, 6.878603939907828, 13.394503618862714, 16.172076823946536, 7.98680455338215, 2.1431667811196435, -0.265816258643991, 4.248005164892988, 11.80914340710262, 18.34643215351687, 15.398753813097944, 12.884596545578033, 6.661889796914567, 9.400983932871922, -2.2204888150709774, 5.137992843372459, 2.093556798962831, 14.472094830687116, 12.592302790749262, 8.096665397104289, 12.98176186475563, 6.02200891782509, 5.476909013494463, 11.274649429401522, 8.891905033497125, 1.7604492209907787, 17.355565302341734, 16.794402190561698, 5.733158218263173, 6.001212894183237, 7.3007451865550355, 10.99081130947398, 7.424387570985898, 9.368788279037965, 7.330622322264265, 7.2987458243054695, 4.172851663016519]}
  out "coherence":cluster{"f0":dbl, "df":dbl, "magnitude":dbl[]}(graph)={"f0"=0.0, "df"=50.000000010186355, "magnitude"=[0.8655427550908729, 0.6162505640214626, 0.31635376401696585, 0.5422115660583012, 0.3802561534716612, 0.031734028900079876, 0.1905426282145167, 0.3023217958135459, 0.5330936629214179, 0.023054247831643435, 0.02574346706386154, 0.16602717795095526, 0.3234868406524516, 0.2878645801144842, 0.6216265767356431, 0.7168813991330111, 0.1414167668065334, 0.16756202028887174, 0.3253071907168125, 0.9999986078103624, 0.9999997232221722, 0.9999982075009771, 0.5134136050775968, 0.6098409075360103, 0.36929262905610566, 0.3036136162728009, 0.6053846929909359, 0.7088061684489761, 0.6927945967893294, 0.28293791273907387, 0.00430175827641113, 0.14887810586464092, 0.32982408070094016, 0.33596340982851175, 0.4452379176877398, 0.4242328058883029, 0.07106846950958379, 0.16677589339081234, 0.03228085895611259, 0.20198261610947732, 0.642616633126286, 0.22339662835474913, 0.47462186758686803, 0.0976755044870434, 0.1386789272057623, 0.15170658109174595, 0.5920519487791328, 0.382206698037567, 0.20623354478469147, 0.644872410201296, 0.4132546929662899, 0.1538673477624695, 0.3831097829495219, 0.40578279983021404, 0.2978977474220297, 0.4805543642592903, 0.3281475016876746, 0.39671588909605493, 0.5727857303220731, 0.11896294337087923, 0.4799105256655794, 0.6124939612073009, 0.12434837761959194, 0.012512754646834058, 0.5463457386691091, 0.5860437664821234, 0.30642963275906215, 0.24993787082797422, 0.2131979679948132, 0.3483733340681083, 0.10127480593713126, 0.4989354603892965, 0.2987461836446398, 0.4050479270406586, 0.3404471990723733, 0.3820433597460375, 0.19077808297565876, 0.08805902303287473, 0.3347473961062396, 0.06318468084373734, 0.4090324129525661, 0.25316973552310224, 0.7289208096503323, 0.09887799753718059, 0.35546122614907005, 0.18936147939995598, 0.30185315209587527, 0.30156512011638287, 0.5056031339402993, 0.18318443406682225, 0.057002671423337564, 0.3233892989765439, 0.5780962990669106, 0.08435711805088285, 0.14209105400757785, 0.05328801628311501, 0.433993572123052, 0.34197891327100766, 0.16242006910148815, 0.33387427804462955, 0.644514469783385, 0.3385148128787685, 0.12669635457818418, 0.17122390124586948, 0.1633668857811028, 0.13965195560726704, 0.7134720139818985, 0.5281608405614847, 0.4211599184133828, 0.34485146677185397, 0.4234926884685013, 0.7504323364829816, 0.015863098228397928, 0.005463144235454591, 0.18389837743514653, 0.26617568573853423, 0.38183380070615935, 0.30092634021471243, 0.11835566982978486, 0.15842660588320795, 0.6452231859074744, 0.3999694548676882, 0.5874118101791463, 0.19915039038784402, 0.2299908954370555, 0.35909073054870955, 0.023546973008010473, 0.2960685742288182, 0.09805537814584689, 0.14514053757337542, 0.022968502054195483, 0.0025964788682141878, 0.16731523778848534, 0.5335291425332752, 0.04076799180671632, 0.226623409565972, 0.13167407462270533, 0.5839799544737672, 0.17394527830296608, 0.9218091864682112, 0.9493992661482701, 0.7044752586054454, 0.07345922037572811, 0.1752384493379958, 0.07118483625067423, 0.047341432603557394, 0.07077368306856324, 0.21662540025540303, 0.6256889398948909, 0.5809245641421333, 0.11872188017365493, 0.5176007670776949, 0.45311584626371865, 0.47343987056674547, 0.35097186049135365, 0.28968365456823897, 0.07551139703682505, 0.005513802369375138, 0.5153164053473143, 0.12986542901710385, 0.3066012614748819, 0.22787787623231653, 0.266146352593897, 0.015370783439815053, 0.027827009686754202, 0.6880774994041288, 0.43702324962769923, 0.3149666426578894, 0.28745694852683623, 0.3461346443883513, 0.033754361784707906, 0.01807264446458822, 0.21468488292702106, 0.13918590468159842, 0.08984022484335748, 0.1922919795626708, 0.22570929226802414, 0.07889215390234233, 0.2336706066847899, 0.42811907961199697, 0.4986697460472068, 0.05026444781292043, 0.03175857897851498, 0.2564930207811104, 0.4252459548563531, 0.38135199546258536, 0.2636580383555316, 0.24875975603833572, 0.39862239259826815, 0.13217455026153016, 0.21977751236611998, 0.11750748507040093, 0.1602538637019939, 0.20030827799357404, 0.3478952615016765, 0.07045313783079123, 0.20438175292211988, 0.24447985581356002, 0.7234470669617769, 0.049359529613360896, 0.048807818698340305, 0.31585931916524196, 0.023199871172321772, 0.4203741448256027, 0.557746576813861, 0.07277593225185097, 0.0637538363656712, 0.3184815791715112, 0.5325982652995845, 0.41257304466205175, 0.35552174469388903, 0.12108172024026476, 0.21864255488151452, 0.48886944787262404, 0.7732775641534717, 0.5644354632213061, 0.20237750674562807, 0.4791185670738266, 0.004208150786434777, 0.3839263552689897, 0.5482259717537118, 0.44597918476209264, 0.6157062114257623, 0.7888337202526703, 0.3654073343736904, 0.013227582838577492, 0.16583742025973994, 0.4194949430779467, 0.4603813527405281, 0.12836451198622228, 0.6805036302532341, 0.14602579205289729, 0.2554448580528395, 0.03942924141224595, 0.6119791835916436, 0.15575789219118732, 0.3889150793876282, 0.03890912742568507, 0.018325531022154472, 0.2439738674070251, 0.5538459336965654, 0.24642762015162709, 0.04716808765025454, 0.21986700141202506, 0.13883010276313845, 0.3304878852018393, 0.37536989760132194, 0.5814492890229794, 0.36989474995765986, 0.07803669203560762, 0.3934731566869332, 0.19250673704633015, 0.16182293044900617, 0.13324199637486223, 0.12127106202134719, 0.051834670000965574, 0.29849305282037436, 0.13703937821468057, 0.11551047022320167, 0.4291049732026773, 0.3838339185599867, 0.35439981909020823, 0.2955980343443698, 0.3138897449564, 0.2705049351790173, 0.005623717877336297, 0.01040654747939312, 0.1922418894528511, 0.0599583259078014, 0.12879809225649502, 0.0656690635053047, 0.19175429703169358, 0.3164659741210351, 0.14164908211973934, 0.14859887096180405, 0.1738488610457077, 0.5819562951397562, 0.5664325103325525, 0.20338043758314, 0.30493491973074444, 0.45436353681591196, 0.33833539828310566, 0.4693412666034578, 0.45071494233384407, 0.380052825751858, 0.34432629879195886, 0.6194971851061014, 0.3158053544013165, 0.21498313796095703, 0.26525368736687605, 0.06380608987427429, 0.626608774544854, 0.40512772271306513, 0.10355822390195164, 0.12008602461595697, 0.25518629434285595, 0.04261419758493891, 0.10595552617601142, 0.3276601914067259, 0.20414006053344683, 0.3161811126214504, 0.0234555751553772, 0.5162019361439998, 0.23351681599145163, 0.2840602602757372, 0.2660249986813234, 0.05712164960550652, 0.4338767194739849, 0.05410248411035101, 0.2916709631448864, 0.28525184793886255, 0.2382884791543303, 0.06689891131653097, 0.16140856803129452, 0.2415481720626587, 0.18248053801280373, 0.09297099361497554, 0.04907733329968905, 0.1005717844557495, 0.2503736003852846, 0.4525224973976457, 0.29007323816466085, 0.5310896254034392, 0.5883436921422014, 0.1792383136543668, 0.50323851819285, 0.48969193339899875, 0.26275159213309085, 0.20770318186853728, 0.33485863991545367, 0.16071879377950724, 0.029666750511972356, 0.25627741493750883, 0.2988121842878775, 0.2893079434770271, 0.14166082781229744, 0.013400016828320515, 0.06621380835017811, 0.25569608622926404, 0.1512538310044213, 0.3378018924834186, 0.23016375912788786, 0.3161362635175713, 0.13498904779660487, 0.24558035484412527, 0.5286879007760196, 0.6046233680958671, 0.24355983717696972, 0.283228650849774, 0.26348740539833043, 0.33619220912267284, 0.2943529139028501, 0.7521229000043196, 0.2836502971233672, 0.17287728583803383, 0.027718006508690076, 0.39856109870069784, 0.09279507157449611, 0.2844208689127284, 0.08558219925930341, 0.21265548262530712, 0.07338584383773593, 0.3708378740674345, 0.4102290189015152, 0.08061331896175698, 0.7238058631115837, 0.1228766538044879, 0.3938135507163275, 0.03237009216822793, 0.5603108699023117, 0.15543687072260154, 0.09709720226881816, 0.22246870451092685, 0.38974946400412197, 0.6120329324436461, 0.42828750180089625, 0.5059875305828248, 0.3265706300402723, 0.5197706151755462, 0.06862217726784728, 0.5877508570613182, 0.41104352977004593, 0.000356106567203599, 0.1620201937509784, 0.13662079480379463, 0.04316468182622781, 0.6821683851469625, 0.4791494552348316, 0.06205734070227232, 0.06037483177933296, 0.06905300787145308, 0.1784228012792312, 0.5720743691830485, 0.09628960782467037, 0.40131570629934527, 0.34100623200609786, 0.23079107041422417, 0.36794150367390355, 0.5299335266609596, 0.4832623353456088, 0.2803868008964997, 0.29482666123519746, 0.21245287051381354, 0.2689983604502641, 0.3875325064830838, 0.42293299512163623, 0.45897001678166033, 0.19755023832325982, 0.2728632189010105, 0.6351019311213865, 0.09216390791537116, 0.563708449634058, 0.002661157144580259, 0.27804714354729204, 0.04713557716097813, 0.21375908437832436, 0.24883915050705996, 0.5790196093732538, 0.520065615547787, 0.2452959900603012, 0.1928971818222056, 0.15291678319921836, 0.36553374542544237, 0.22846104106356846, 0.00479430209971323, 0.1609320717493416, 0.33146268872752804, 0.5306964708210952, 0.18012987418227414, 0.1936902133547007, 0.700046180431597, 0.3868259105838294, 0.15191896141601335, 0.3872062503510825, 0.4866102170329646, 0.1464163566741272, 0.0022382081701962614, 0.28095899392930357, 0.22322974522096906, 0.0684715393125578, 0.4185097530501208, 0.17747816944255843, 0.16505638865098016, 0.05092940653919975, 0.30934803727576093, 0.01630112168136596, 0.024648573112518404, 0.08895826093165222, 0.05065403251206254, 0.028963772146239915, 0.28036570353845436, 0.08902917672547538, 0.18206614802635107, 0.1648379886051829, 0.2644379276687437, 0.24974061509299247, 0.6891101636313678, 0.7390912214733207, 0.470251360026719, 0.34146865103327223, 0.06830484067514939, 0.24821234492919947, 0.485231678368001, 0.13691028190904186, 0.11375904041739425, 0.5046932885664722, 0.4019954235214659, 0.25309825777915146, 0.05565119527868788, 0.03868409798852842, 0.14729430873996147, 0.5860947787161458, 0.2464822692450005, 0.4878806869592468, 0.6692949155317534, 0.462748568011234, 0.3652897547523206, 0.061175591208240565, 0.2095178714709747, 0.05899486843065817, 0.6363691100257689, 0.8283803086844894, 0.5892187416812861, 0.4540226241724836, 0.1672650517373276, 0.20156110266359564, 0.34600013893359155, 0.2493174291801288, 0.0396601497563084, 0.563743639351697, 0.7101308227120398, 0.35906653484676854, 0.2477460086718607, 0.23369471314331952, 0.38864975208323244, 0.33717278660981775, 0.3081431539429594, 0.4423647181320473, 0.4464140191544251, 0.21674863453232113]}
  in  "desired units":T9={"THD units"=enum."%", "harmonic component amplitude units"=enum."EU peak", "detected fundamental amplitude units"=enum."EU peak"}
  in  "maximum harmonic":i32=-1
  in  "harmonics to visualize":i32[](array[numeric])=[-1]
  out "expected fundamental frequency [Hz]":dbl=1000.0 format="%.2f"
  out "actual maximum harmonic":i32=24
  out "THD":dbl=0.5255530851064686 format="%.2f"
  out "detected fund. amp.":dbl=0.4482732881746804 format="%.5f"
  out "detected fund. freq. [Hz]":dbl=1000.0480977732343 format="%.2f"
  out "THD(%)":dbl(graph)=0.5255530851064686
  out "fft":cluster{"f0":dbl, "df":dbl, "magnitude":dbl[]}(graph)={"f0"=0.0, "df"=50.000000010186355, "magnitude"=[-49.550436026747605, -45.749287306360415, -53.36006996929462, -70.30950780535235, -70.9243853905227, -70.636468228137, -80.04167938111196, -76.318751863545, -75.01818724956263, -87.60585116004506, -89.69236540900582, -84.33259568109861, -78.84781783779458, -79.83716954945413, -79.97268572654292, -80.76857496666504, -78.95002468537852, -84.35793521738866, -76.357502829623, -16.004511450443523, -9.98429274821412, -15.99426056011656, -71.2924060770297, -77.82445851043313, -74.92104140869999, -75.5515686017999, -73.40763479753306, -66.24461005797812, -69.9880337911179, -74.35089176454494, -74.35115004129399, -76.64885780390327, -76.9370780440231, -83.18573138471494, -88.76437168827667, -81.4236319264927, -85.73146800810322, -81.83025126661218, -83.2803228330879, -61.88772701189951, -55.91310371312449, -61.528148209078765, -82.8853478215892, -92.42931513143856, -95.21330465722983, -90.14600452102137, -87.52250131598768, -89.9309237636491, -93.06952313014305, -88.73100805891443, -87.97078967553398, -97.28842588259442, -115.04607806200559, -93.78603715290919, -96.47932232708703, -87.71621427126242, -85.52942024977612, -89.18349024657834, -94.9383059168641, -77.37522585116844, -71.64845390576524, -77.7025404755032, -95.65915916194982, -120.79466807428025, -94.17219436450378, -88.4215141896823, -87.0329413672739, -88.28005719307342, -92.42529946012252, -93.81098694318709, -93.80775410930534, -97.20566593400717, -93.67580077029916, -89.90042707183201, -86.95056331332722, -89.40455807579548, -102.11022731450223, -95.60173470211907, -97.66374047942318, -88.94882890460016, -86.34533062908517, -84.29052581589325, -88.47055959193035, -101.93605007871611, -94.4173738840408, -95.19917851780852, -99.95817732578898, -106.16981845041124, -93.14297082231619, -92.54877138488602, -100.85995864006856, -97.77435540231556, -109.15398934849448, -94.43915059538998, -92.24856180006384, -91.13155171820387, -91.25403532428868, -105.1592822182069, -96.24272940477906, -87.62678922925718, -84.9440912011017, -93.74405326148805, -90.016028502225, -91.77060086484965, -97.03267862654585, -96.01642916234886, -115.48711636245842, -93.01933645592402, -87.33086822946768, -87.14243732599122, -96.07440699238799, -99.60688105373876, -92.38187740754121, -89.87161827367247, -94.08712097525341, -102.09094984656059, -104.30483775480901, -102.52433231797595, -105.37734282049217, -100.22160347910332, -95.12950207807921, -100.1302071685659, -99.06804471711882, -95.01647857765622, -95.28328646849138, -94.86669486094371, -98.86100991373745, -102.57706798879076, -108.39125460444869, -98.43951071719675, -99.67108519975001, -106.5721161253124, -100.29106164830154, -95.62267961075705, -94.13934585469997, -95.78774321230831, -95.50990579214344, -101.97006364198285, -98.47141331268261, -96.24702187884313, -92.81877362431004, -94.64522598626334, -99.70048838900725, -106.85884111051494, -99.07245228796194, -101.58607031819201, -108.41312055533884, -99.51412405168021, -92.00431005299959, -91.77265840243372, -100.33685554485523, -100.53329238886423, -98.5803872133474, -98.74059148987055, -98.98436243926457, -101.96270532847237, -97.77434029459181, -96.11561815572982, -98.23367164445796, -104.03637148403753, -99.61204780354689, -100.3917093309329, -100.93956783705671, -105.98365552742456, -110.66522155526164, -107.20649600273033, -98.71673598612246, -96.08684267697396, -95.09452098924052, -100.22540716480579, -108.12252688061747, -108.90853467828248, -104.22628734085342, -101.21554058930577, -105.80060525878208, -107.2884836740393, -103.62663036061005, -99.55378116179772, -110.2198309472554, -100.64807269073958, -102.70325519159948, -111.26365513700036, -101.10668166401518, -106.12777053298427, -105.98098816891337, -105.95990544920645, -100.63250424575577, -99.73495121044692, -97.01192061340214, -100.11966249293609, -97.28973698446595, -96.53664698634606, -101.97011614576438, -105.48182953310302, -95.6201146367392, -98.83650442252025, -102.12176162331241, -103.8644166375871, -103.87885782328414, -96.88185279228611, -101.07328034556744, -103.1641907181297, -98.60107878758865, -99.07382546674884, -101.85132023012054, -101.72214658354848, -101.40710964352729, -102.24939284981232, -100.39018178308177, -105.3169904876076, -96.73798807123833, -104.6377736104872, -100.49232540986387, -99.67887788954397, -98.68019350076924, -100.57486157153187, -118.31788905027923, -99.09170482070829, -96.55816253054067, -93.10275086606129, -93.92678803255447, -103.65445489846462, -100.68329184209577, -95.46374432505411, -100.09156637173572, -119.75334757967633, -103.83895332070531, -97.91439814670981, -100.14328599428602, -102.37652739339582, -97.05012122445495, -98.78441073717403, -106.46216130591941, -103.78124777892552, -97.56828934132099, -98.30812119039919, -106.38467150417492, -108.91248733157396, -110.24732804761658, -99.93675559392435, -96.22025462101915, -100.63146041955565, -108.8469166683519, -102.98524805929296, -100.7011517757447, -96.8076038140279, -100.73141909710037, -105.59232969729848, -101.85490742777017, -109.93519203335886, -106.28216286708812, -107.85238482832291, -108.94211714268492, -109.11966901034369, -103.61755268353073, -108.11852152422978, -102.78404032133749, -98.25650613236408, -99.57606302006926, -102.80638169311892, -108.3759488997321, -103.42818343283915, -97.05004251920005, -96.22470088845715, -101.67033894868098, -112.58572219763599, -113.19031655992643, -108.20147787634424, -108.82798990976252, -102.2236480388791, -95.57247191868586, -96.65751151035218, -103.47093340534038, -118.60185455970102, -102.77673311402543, -119.10403152172827, -100.73814988795155, -107.03008641378858, -110.36567083261369, -103.81092733881049, -102.08327211002347, -112.6521007037525, -133.42262063775132, -105.75193616535739, -103.3446051421192, -104.43949625932328, -112.00519689092962, -102.41091750580512, -104.20201167452952, -106.65971089414379, -101.59506693421646, -103.41555281625061, -108.62808895252093, -108.0407684916797, -105.21076526080401, -103.05278785895237, -109.94493950788572, -112.32773740094608, -118.87348510759053, -104.18400687711525, -102.69535121061278, -109.16900297787134, -105.29273913222895, -97.44247192548471, -96.01806440431238, -96.93652794736616, -98.00353128375492, -102.06404173817675, -110.20319061055801, -104.48124877112832, -106.34265020620057, -96.31741533260808, -97.55305262250019, -104.60328541366462, -107.21119851197858, -115.36232265281471, -113.52996389664852, -117.46541607919106, -107.65137526072434, -100.12841546926639, -99.05816941374, -106.1821010885723, -100.4283173471409, -99.43342714012638, -105.73463621845137, -103.3985322900223, -108.06406472605437, -110.87428086755843, -106.94115483597756, -105.46897363070585, -103.78137388746836, -106.46241618120543, -105.23597464060883, -105.41845854256357, -107.14436146193856, -104.58512823311055, -107.41006929681568, -111.41857627238379, -109.64819585102154, -105.16089663384182, -103.74645584254407, -109.11119356498975, -109.73029797778864, -115.31193824118844, -108.49674859289158, -102.6656304067218, -105.40420006788592, -105.16225128155547, -98.04242953357297, -105.56899590099752, -108.66344251093523, -104.49854061140984, -101.7691873193162, -104.60771603896373, -104.51457670341007, -100.19399933903024, -98.30342753116007, -98.20802779359182, -103.6847764404522, -123.25769640922162, -109.74195021548692, -111.70120394645436, -106.5309728629515, -102.15454593292478, -107.075450703598, -105.72523587888946, -111.86346323622503, -107.73926105470188, -107.38008972281493, -105.86119743955007, -125.8840253764892, -112.72686179775597, -106.41246324813663, -103.2240688868945, -102.6495194754152, -104.276378888983, -109.63612127460821, -120.03266434027361, -114.05025057696443, -103.84974706078766, -98.67513083885511, -97.64204634099777, -100.63113185896057, -112.10639950689504, -106.97026167279573, -104.09158121927112, -100.41433329582544, -101.0530130849931, -108.70068943746705, -114.39866021070782, -117.61412650417255, -110.47919717840529, -110.5028182368186, -111.47904496217848, -101.78880278323227, -100.87777472477896, -102.72744070256593, -105.71635322716956, -102.56381001969973, -108.60509017924089, -105.7245485150497, -111.21717929192354, -112.1490233319694, -106.76204052693637, -107.34714478825309, -106.59666911877403, -104.47779710954593, -107.54548557709268, -116.11022475944426, -107.49788635413017, -106.54878370453585, -114.95475849341021, -121.32146888310864, -115.87767407298753, -105.83235072034425, -106.87017035483399, -109.75640698772227, -105.3210968952874, -104.01739889094532, -102.65946881102434, -106.93641723534816, -108.24527332277339, -107.56986063984783, -110.91994060466234, -116.40917819338165, -107.71830760514985, -114.65087131704428, -104.27504468673911, -104.50576967303179, -105.89090146754373, -108.56273645308674, -109.5284365158821, -119.94947556075181, -111.48407622298762, -109.66954056523949, -107.26589805950044, -110.60670522292722, -106.8862137344033, -102.95925349389434, -99.16310910214918, -97.7065214696648, -102.80969069759954, -117.0877885318943, -116.84599635783798, -112.3950496405109, -108.96699367634983, -105.90571426828322, -106.73751230481193, -108.11494254625428, -106.7593899296372, -102.89224101558403, -103.21724971588279, -110.08484482626616, -108.34151990247497, -105.75572212666546, -109.91897258573488, -105.72188899825149, -99.49109543909707, -100.95745836811412, -104.77045103486928, -106.51896751119602, -109.92430603679401, -110.69749166132368, -107.58045793531593, -108.32172191483002, -111.60293210545814, -104.24901894750775, -108.89869012791438, -107.97859151064569, -109.37465993891662, -108.63899624070727, -106.38651044702607, -102.10394008115946, -102.66080302797951, -104.72400032911013, -112.7870478848595, -112.2817525593212, -124.04202892984287, -117.3361569915993, -119.16402172325485, -105.8355372173945, -105.34080919106829, -106.01406048377783, -103.23823477980363, -111.38010917939985, -111.75006261028422, -108.25099485837099, -106.40365272974167, -109.3954790519558, -107.11418251901763, -105.73291473563617, -115.64993532535395, -111.33076248643819, -111.7906685070813, -111.66709363777663, -112.1476836883216, -111.47192423857538, -112.96970201516446, -116.17215582808917, -112.40614670941676]}
  in  "dB On (T)":bool=TRUE
  out "coherence 2":dbl(graph)=999.9997232221722
  out "COH":dbl=999.9997232221722 format="%.10f"
  in  "frequency":dbl=1000.0
  in  "stop":bool
  out "loop time(ms)":u32=19
  out "XY Graph":cluster{dbl[], dbl[]}[](graph)=[{[0.021, 0.041, 0.07, 0.08700000000000001, 0.10600000000000001, 0.125, 0.144, 0.16299999999999998, 0.18799999999999997, 0.20699999999999996, 0.22699999999999995, 0.24499999999999994, 0.26299999999999996, 0.285, 0.305, 0.323, 0.34500000000000003, 0.36400000000000005, 0.38300000000000006, 0.4060000000000001, 0.4250000000000001, 0.4440000000000001, 0.46500000000000014, 0.48500000000000015, 0.5050000000000001, 0.5240000000000001, 0.5440000000000002, 0.5630000000000002], [0.0, 0.0, 0.5127202121287527, 0.5468147178491373, 0.5113935934065261, 0.5152460422350947, 0.5067297223462083, 0.5642839414237978, 0.5746230723002935, 0.545398761909948, 0.5338370932650872, 0.551146395387674, 0.5719764653070627, 0.5375454545895423, 0.537446460172108, 0.5808316642168437, 0.5322047145448163, 0.542195941406813, 0.5587662684664381, 0.535636496263525, 0.5091814361274755, 0.530595639527823, 0.5291564969244456, 0.5460569136668927, 0.5432199651402557, 0.5429647634305357, 0.513659110796227, 0.5255530851064686]}, {[0.021, 0.041, 0.07, 0.08700000000000001, 0.10600000000000001, 0.125, 0.144, 0.16299999999999998, 0.18799999999999997, 0.20699999999999996, 0.22699999999999995, 0.24499999999999994, 0.26299999999999996, 0.285, 0.305, 0.323, 0.34500000000000003, 0.36400000000000005, 0.38300000000000006, 0.4060000000000001, 0.4250000000000001, 0.4440000000000001, 0.46500000000000014, 0.48500000000000015, 0.5050000000000001, 0.5240000000000001, 0.5440000000000002, 0.5630000000000002], [0.0, 0.0, 999.682013442989, 999.7878541951989, 999.8776584092046, 999.9330210698104, 999.9651620975692, 999.980435234377, 999.9900838673566, 999.9945241229253, 999.9972513707472, 999.9984267325082, 999.9988412163327, 999.9989324852683, 999.9993868801159, 999.9996654435182, 999.9998324019856, 999.9992499916435, 999.9994172112486, 999.9996056577829, 999.9997176651168, 999.9998479732699, 999.9998444777252, 999.9999087548579, 999.9997587442951, 999.9998355440711, 999.9998944570908, 999.9997232221722]}]
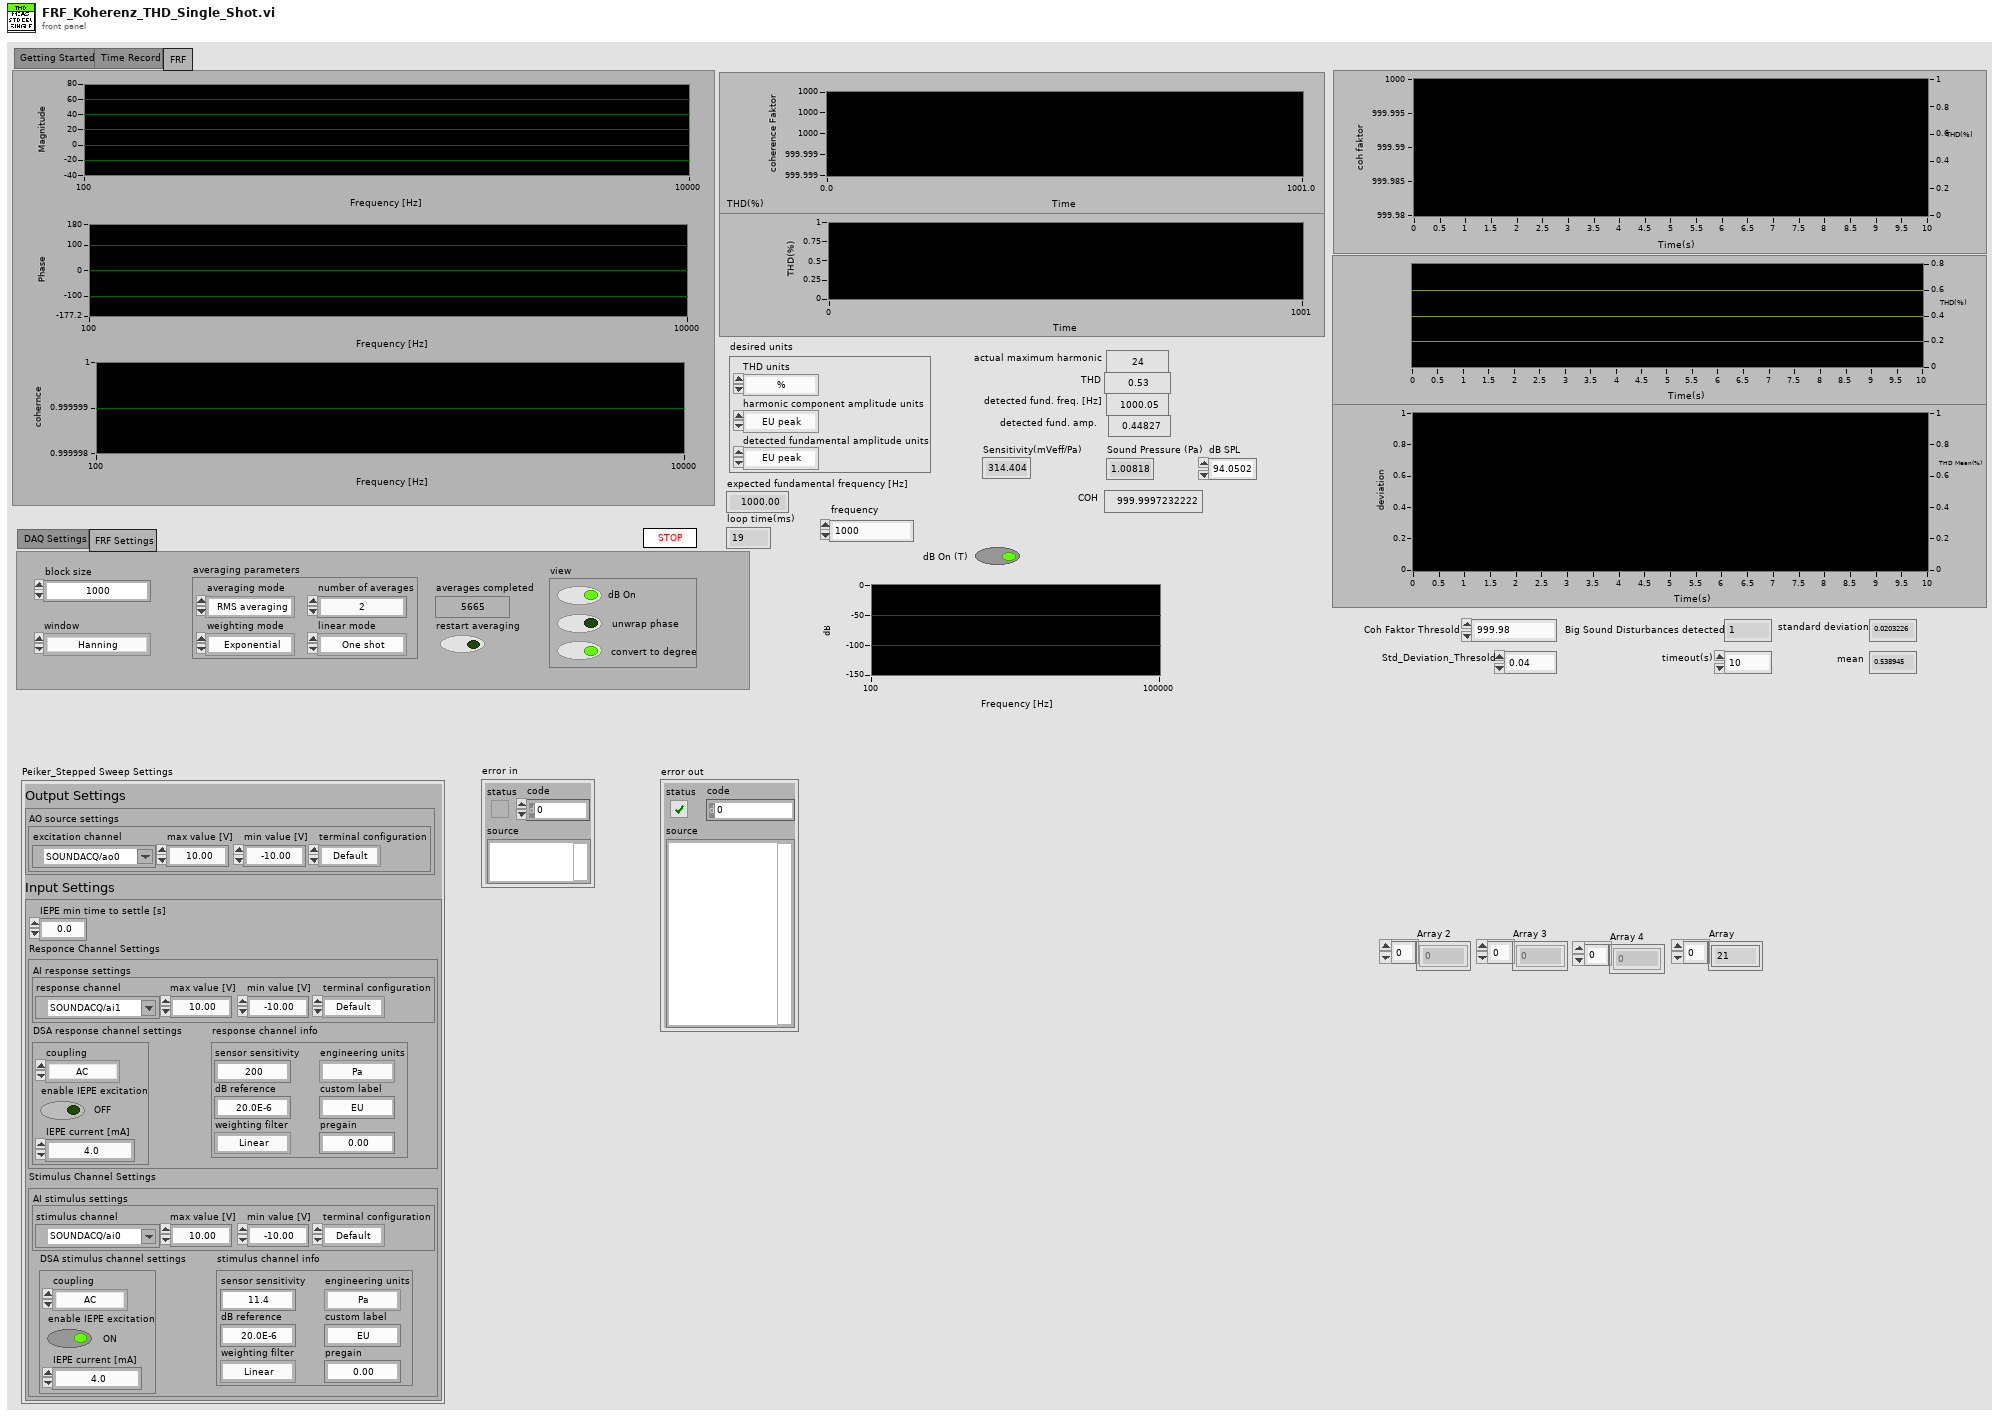
[diagram p1: front panel]
types:
  T1 = typedef "Peiker_Stepped Sweep Settings.ctl" = cluster{"Input Settings":cluster{"IEPE min time to settle [s]":dbl, "Responce Channel Settings":cluster{"DSA response channel settings":T2, "response channel info":T3, "AI response settings":cluster{"response channel":tag, "max value [V]":dbl, "min value [V]":dbl, "terminal configuration":i32}}, "Stimulus Channel Settings":cluster{"AI stimulus settings":cluster{"stimulus channel":tag, "max value [V]":dbl, "min value [V]":dbl, "terminal configuration":i32}, "DSA stimulus channel settings":T2, "stimulus channel info":T3}}, "Output Settings":cluster{"AO source settings":cluster{"excitation channel":tag, "max value [V]":dbl, "min value [V]":dbl, "terminal configuration":i32}}}
  T2 = typedef "svc_DSA Channel Settings.ctl" = cluster{"coupling":i32, "enable IEPE excitation":bool, "IEPE current [mA]":dbl}
  T3 = typedef "svc_Channel Info.ctl" = cluster{"sensor sensitivity":dbl, "engineering units":T4, "dB reference":dbl, "custom label":string, "weighting filter":T5, "pregain":dbl}
  T4 = typedef "svc_Engineering Units Text Ring.ctl" = u16
  T5 = typedef "svc_Weighting Filter Text Ring.ctl" = u16
  T6 = cluster{"averaging mode":enum16{"No averaging", "Vector averaging", "RMS averaging", "Peak hold"}, "weighting mode":enum16{"Linear", "Exponential"}, "number of averages":u32, "linear mode":enum16{"One shot", "Auto restart"}}
  T7 = cluster{"dB On":bool, "unwrap phase":bool, "convert to degree":bool}
  T8 = typedef "svc_Window [Dual FFT].ctl" = u32
  T9 = cluster{"THD units":enum16{"dB", "linear ratio", "%"}, "harmonic component amplitude units":enum16{"EU rms", "EU peak", "EU peak-peak", "dB ref fund"}, "detected fundamental amplitude units":enum16{"EU rms", "EU peak", "EU peak-peak"}}
  T10 = enum16{"uniform white noise", "Gaussian white noise", "periodic random noise", "Chirp"}
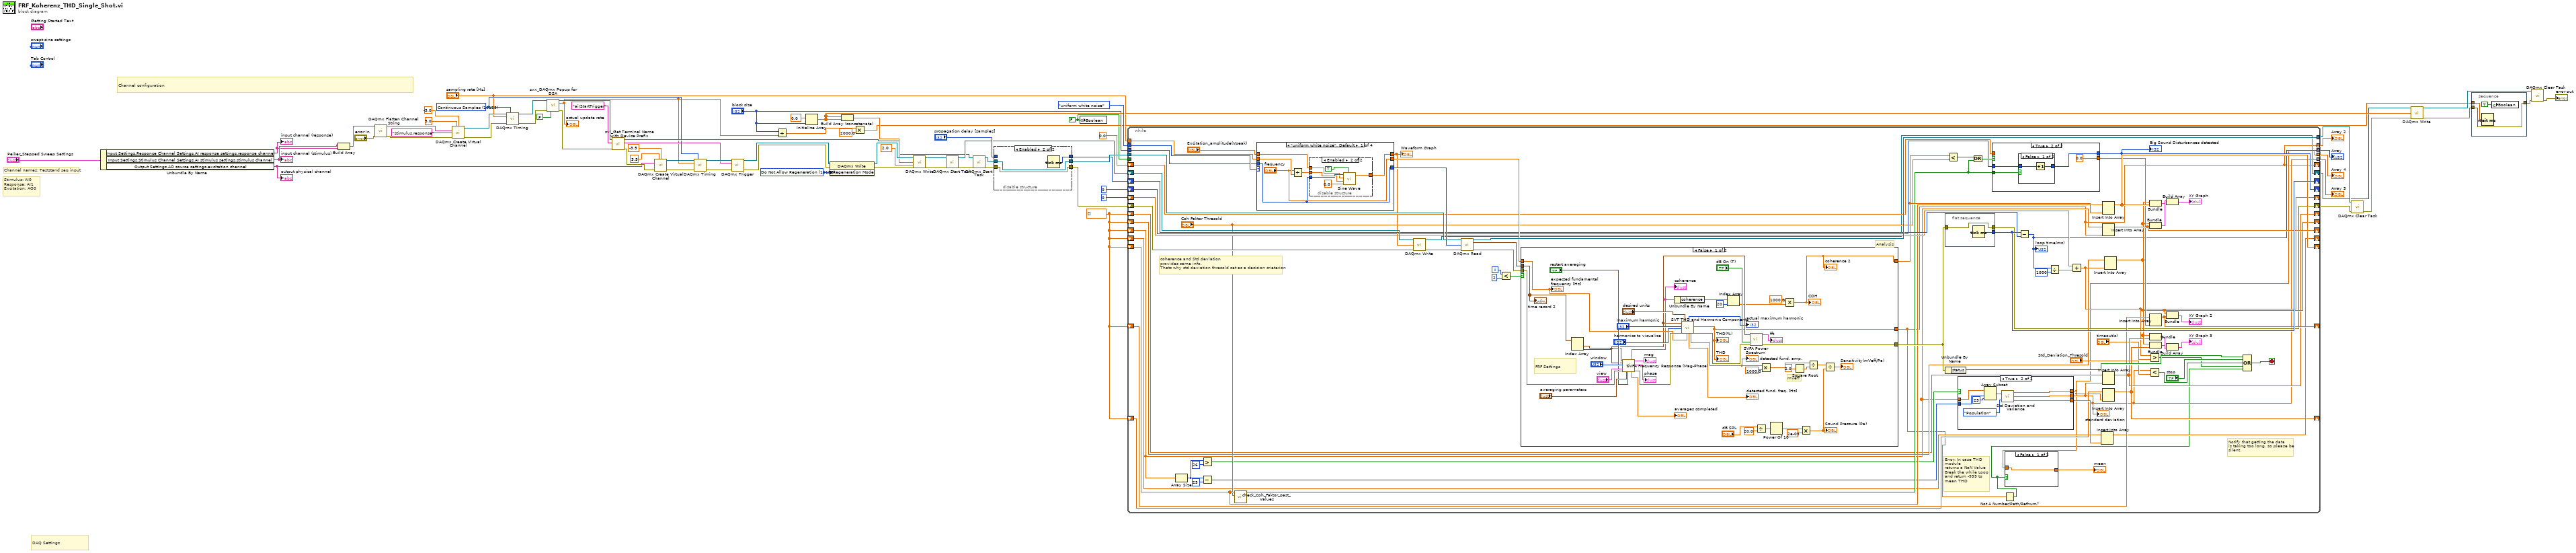
[diagram p0: block diagram]
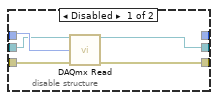
[diagram p2: hidden frame]
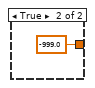
[diagram p3: hidden frame]
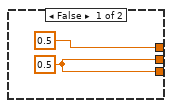
[diagram p4: hidden frame]
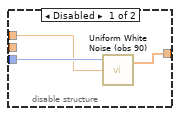
[diagram p7: hidden frame]
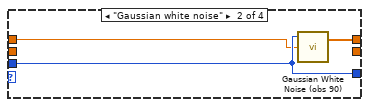
[diagram p8: hidden frame]
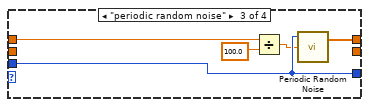
[diagram p9: hidden frame]
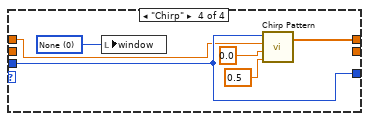
[diagram p10: hidden frame]
diagram:
  w12 = FALSE ("Boolean")
  w17 = dbl[] []
  w60 = 10158 items=["Allow Regeneration"=10097, "Do Not Allow Regeneration"=10158] ("RegenMode")
  w28 = 10123 items=["Finite Samples"=10178, "Continuous Samples"=10123] ("sample mode")
  # "Channel names: Teststand seq input"
  # "Stimulus: AI0\nResponse: AI1\nExcitation: AO0"
  # "Channel configuration"
  # "DAQ Settings"
  n1 = Unbundle By Name("Peiker_Stepped Sweep Settings") -> ("Input Settings.Responce Channel Settings.AI response settings.response channel"=w8:tag, "Input Settings.Stimulus Channel Settings.AI stimulus settings.stimulus channel"=w9:tag, "Output Settings.AO source settings.excitation channel"=w10:tag)
  "input channel (stimulus)" <- w9
  "output physical channel" <- w10
  "input channel (response)" <- w8
  n2 = Build Array(w9, w8) -> (w23:tag[])
  n3 = call <vilib>:"DAQmx Flatten Channel String.vi"("names in"=w23, "error in"="error in") -> ("names out"=w22:string, "error out"=w7:errorcluster)  [unwired: 12 in]
  n4 = call-poly <vilib>:"DAQmx Create Virtual Channel.vi"("maximum value"=5.0, "minimum value"=-5.0, "physical channels"=w22, "name to assign"="stimulus,response", "error in"=w7) -> ("task out"=w40:refnum<k21>, "error out"=w39:errorcluster)  [unwired: 9 in]
  n5 = call-poly <vilib>:"DAQmx Timing.vi"("task/channels in"=w40, "sample mode"=w28, "rate"="sampling rate [Hz]", "error in"=w39) -> ("task out"=w26:refnum<k21>, "error out"=w25:errorcluster)  [unwired: 10 in]
  n6 = call <vilib>:"svx_DAQmx Popup for DSA.vi"("task in"=w26, "error in (no error)"=w25, "interactive configuration dialog"=FALSE) -> ("task out"=w35:refnum<k21>, "actual sample rate"=w24:dbl, "error out"=w34:errorcluster)  [unwired: 10 in]
  "actual update rate" <- w24
  n7 = call <vilib>:"svl_Get Terminal Name with Device Prefix.vi"("error in (no error)"=w34, "local terminal name"="ai/StartTrigger", "task/channels in"=w35) -> ("error out"=w38:errorcluster, "terminal name with device prefix"=w27:tag, "task out"=w37:refnum<k21>)  [unwired: 6 in]
  n8 = call-poly <vilib>:"DAQmx Create Virtual Channel.vi"("maximum value"=3.5, "minimum value"=-3.5, "physical channels"=w10, "error in"=w38) -> ("task out"=w70:refnum<k21>, "error out"=w69:errorcluster)  [unwired: 10 in]
  n9 = call-poly <vilib>:"DAQmx Timing.vi"("task/channels in"=w70, "sample mode"=w28, "rate"=w24, "error in"=w69) -> ("task out"=w68:refnum<k21>, "error out"=w67:errorcluster)  [unwired: 10 in]
  n10 = call-poly <vilib>:"DAQmx Trigger.vi"("task/channels in"=w68, "source"=w27, "error in"=w67) -> ("task out"=w64:refnum<k21>, "error out"=w63:errorcluster)  [unwired: 11 in]
  n11 = Divide(x="block size", y=w24) -> (x/y=w47:dbl)
  n12 = Initialize Array(0.0 ("element"), "block size") -> (w52:dbl[])
  n13 = property class="DAQmx Write"(reference=w64, error in=w63, "Regeneration Mode"=w60) -> (reference out=w62:refnum<k21>, error out=w61:errorcluster)
  n14 = Build Array (concatenate)(w52, w52) -> (w45:dbl[])
  n15 = Multiply(x=w47, y=2000.0) -> (x*y=w44:dbl)
  n16 = call-poly <vilib>:"DAQmx Write.vi"("task/channels in"=w62, "data"=w45, "timeout"=2.0 ("Wirite Timeout"), "error in"=w61) -> ("task out"=w66:refnum<k21>, "error out"=w65:errorcluster)  [unwired: 9 in, 1 out]
  n17 = call <vilib>:"DAQmx Start Task.vi"("task/channels in"=w66, "error in"=w65) -> ("task out"=w56:refnum<k21>, "error out"=w36:errorcluster)  [unwired: 12 in]
  n18 = call <vilib>:"DAQmx Start Task.vi"("task/channels in"=w37, "error in"=w36) -> ("task out"=w41:refnum<k21>, "error out"=w42:errorcluster)  [unwired: 12 in]
  n19 = disable-structure shown="Enabled" {
    disable-tunnel: "propagation delay [samples]" -> [w77 _]
    disable-tunnel: [w76 w80] -> w55
    disable-tunnel: [w75 w79] -> w54
    disable-tunnel: w42 -> [w74 w79]
    disable-tunnel: w41 -> [w73 w80]
    disable-tunnel: [_ w78] -> w14
    frame Disabled {
      n20 = call-poly <vilib>:"DAQmx Read.vi"("task/channels in"=w73, "number of samples per channel"=w77, "error in"=w74) -> ("task out"=w76:refnum<k21>, "error out"=w75:errorcluster)  [unwired: 10 in, 1 out]
    }
    frame Enabled {
      n21 = Tick Count (ms)() -> (millisecond timer value=w78:u32)
    }
  }
  n22 = global write "THD_Mess_Status.vi" "Boolean"(w12) -> ()
  n23 = while {
    tunnel: "block size" -> [w152]
    tunnel: T10."uniform white noise" ("excitation") -> [w153]
    tunnel: [w141] -> w59
    tunnel: w55 -> [w143]
    tunnel: "sampling rate [Hz]" -> [w139]
    shift-right: [w136] -> _
    shift-left: w14 -> [w135]
    shift-right: [w98] -> _
    shift-left: w17 -> [w133]
    shift-right: [w132] -> _
    shift-left: w17 -> [w109]
    shift-right: [w124] -> _
    shift-left: w17 -> [w115]
    shift-right: [w89] -> _
    shift-left: 0 -> [w128]
    shift-right: [w119] -> _
    shift-left: w17 -> [w122]
    shift-right: [w120] -> _
    shift-left: 0 -> [w121]
    shift-right: [w82] -> _
    shift-left: 0.0 ("THD") -> [w112]
    shift-right: [w97] -> _
    shift-left: w17 -> [w106]
    shift-right: [w96] -> _
    shift-left: w17 -> [w105]
    shift-right: [w107] -> _
    shift-left: w17 -> [w104]
    tunnel: [w93] -> w16 mode=indexing
    shift-right: [w92] -> w15
    shift-left: w56 -> [w144]
    tunnel: w12 -> [_]
    shift-right: [w86] -> w4
    shift-left: w54 -> [w142]
    tunnel: [w82] -> w3 mode=indexing
    tunnel: [w85] -> w2 mode=indexing
    tunnel: [w84] -> w1 mode=indexing
    i -> [w155]
    stop <- w150 stop-if-true
    # "coherence and Std deviation \nprovides same info.\nThats why std deviation thresold set as a decision crieterion"
    # "Error: In case THD \nmodule \nreturns a NaN Value\nBreak the while Loop \nand return -999 to \nmean THD"
    # "Notify that getting the data \nis taking too long, so please be \nsilent."
    # "Analysis"
    n24 = Array Size(array=w109) -> (size(s)=w102:i32)
    n25 = Greater?(x=w102, y=26) -> (0:w110:bool)
    n26 = Subtract(x=w102, y=25) -> (x-y=w103:i32)
    n27 = call "check_Coh_Faktor_past_Values.vi"("Coh Faktor Thresold in"="Coh Faktor Thresold", "Array"=w115) -> ("Boolean"=w113:bool)  [unwired: 9 in]
    n28 = case shown="\"uniform white noise\", Default" w153 {
      tunnel: [w179 w196 w201 w207] -> w134
      tunnel: w152 -> [w184 w195 w200 w206]
      tunnel: [w184 w195 w200 w206] -> w145
      tunnel: "Excitation_amplitude(Vpeak)" -> [w183 w194 w198 w202]
      tunnel: w139 -> [w181 _ _ _]
      tunnel: ["frequency" _ _ _] -> w138
      frame "uniform white noise", Default {
        n29 = Divide(x="frequency", y=w181) -> (x/y=w182:dbl)
        n30 = disable-structure shown="Enabled" {
          disable-tunnel: [w187 w193] -> w179
          disable-tunnel: w184 -> [w186 w190]
          disable-tunnel: w183 -> [w185 w188]
          disable-tunnel: w182 -> [_ w191]
          frame Disabled {
            n31 = call <vilib>:"Uniform White Noise (obs 90).vi"("amplitude"=w185, "samples"=w186) -> ("uniform white noise"=w187:dbl[])  [unwired: 1 in, 1 out]
          }
          frame Enabled {
            n32 = call <vilib>:"Sine Wave.vi"("samples"=w190, "amplitude"=w188, "frequency"=w191, "phase in"=0.0, "reset phase"=TRUE) -> ("sine wave"=w193:dbl[])  [unwired: 2 out]
          }
        }
      }
      frame "Gaussian white noise" {
        n33 = call <vilib>:"Gaussian White Noise (obs 90).vi"("standard deviation"=w194, "samples"=w195) -> ("Gaussian noise pattern"=w196:dbl[])  [unwired: 1 in, 1 out]
      }
      frame "periodic random noise" {
        n34 = Divide(x=w198, y=100.0) -> (x/y=w197:dbl)
        n35 = call <vilib>:"Periodic Random Noise.vi"("spectral amplitude"=w197, "samples"=w200) -> ("periodic random noise"=w201:dbl[])  [unwired: 1 in, 1 out]
      }
      frame "Chirp" {
        w205 = T8 0 items=["None"=0, "Hanning"=1, "Hamming"=2, "Blackman-Harris"=3, "Exact Blackman"=4, "Blackman"=5, "Flat Top"=6, "4 Term B-Harris "=7, "7 Term B-Harris"=8, "Low Sidelobe"=9, "Force - Exponential"=10, "Blackman Nuttall"=11, "Triangle"=30, "Bartlett-Hanning"=31, "Bohman"=32, "Parzen"=33, "Welch"=34, "Kaiser"=60, "Dolph-Chebyshev"=61, "Gaussian"=62] ("window")
        n36 = local write "window"(w205) -> ()
        n37 = call <vilib>:"Chirp Pattern.vi"("f2"=0.5, "f1"=0.0, "amplitude"=w202, "samples"=w206) -> ("Chirp Pattern"=w207:dbl[])  [unwired: 1 out]
      }
    }
    "Waveform Graph" <- w134
    n38 = call-poly <vilib>:"DAQmx Write.vi"("task/channels in"=w144, "data"=w134, "error in"=w142) -> ("task out"=w92:refnum<k21>, "error out"=w148:errorcluster)  [unwired: 10 in, 1 out]
    n39 = call-poly <vilib>:"DAQmx Read.vi"("task/channels in"=w143, "number of samples per channel"=w145, "error in"=w148) -> ("task out"=w141:refnum<k21>, "data"=w146:waveform(dbl)[], "error out"=w147:errorcluster)  [unwired: 10 in]
    n40 = Less?(x=w155, y=2) -> (x < y?=w154:bool)
    n41 = case shown="False" w154 {
      tunnel: w147 -> [w249 w250]
      tunnel: w146 -> [w241 _]
      tunnel: [w228 w250] -> w137
      tunnel: w138 -> [w233 _]
      tunnel: [w222 _] -> w125
      tunnel: [w221 _] -> w82
      frame False {
        # "FRF Settings"
        # "mVeff"
        n42 = Index Array(array=w241) -> (element #1=w240:waveform(dbl), element #2=w232:waveform(dbl))  [unwired: 2 in]
        n43 = call-poly <vilib>:"SVFA Frequency Response (Mag-Phase).vi"("stimulus signal X [EUx]"=w240, "response signal Y [EUy]"=w232, "window"="window", "view"="view", "error in (no error)"=w249, "averaging parameters"="averaging parameters", "restart averaging (F)"="restart averaging") -> ("coherence"=w227:cluster{"f0":dbl, "df":dbl, "coherence":dbl[]}, "averages completed"=→"averages completed":dbl, "magnitude [dB EUy/EUx]"=→"mag":cluster{"f0":dbl, "df":dbl, "magnitude":dbl[]}, "phase [degrees]"=→"phase":cluster{"f0":dbl, "df":dbl, "phase":dbl[]}, "error out"=w234:errorcluster)  [unwired: 4 in, 4 out]
        "coherence" <- w227
        n44 = Unbundle By Name(w227) -> ("coherence"=w226:dbl[])
        n45 = call-poly <vilib>:"SVT THD and Harmonic Components.vi"("scaled signal [EU]"=w232, "maximum harmonic"="maximum harmonic", "harmonics to visualize"="harmonics to visualize", "error in (no error)"=w234, "desired units"="desired units", "expected fundamental frequency [Hz]"=w233) -> ("actual maximum harmonic"=→"actual maximum harmonic":i32, "detected fundamental\nfrequency [Hz]"=→"detected fund. freq. [Hz]":dbl, "detected fundamental\namplitude"=w220:dbl, "THD"=w221:dbl, "error out"=w229:errorcluster)  [unwired: 6 in, 3 out]
        "THD" <- w221
        "detected fund. amp." <- w220
        "THD(%)" <- w221
        n46 = Index Array(array=w226, index=20) -> (element=w224:dbl)
        n47 = call-poly <vilib>:"SVFA Power Spectrum.vi"("scaled signal [EU]"=w232, "dB On (T)"="dB On (T)", "error in (no error)"=w229) -> ("power spectrum [dB EU]"=→"fft":cluster{"f0":dbl, "df":dbl, "magnitude":dbl[]}, "error out"=w228:errorcluster)  [unwired: 11 in, 4 out]
        n48 = Divide(x="dB SPL", y=20.0 ("x")) -> (x/y=w212:dbl)
        n49 = Multiply(x=w220, y=1000.0 ("x")) -> (x*y=w218:dbl)
        n50 = Power Of 10(x=w212) -> (10^x=w211:dbl)
        n51 = Multiply(x=1000.0, y=w224) -> (x*y=w222:dbl)
        "coherence 2" <- w222
        "COH" <- w222
        n52 = Square Root(x=2.0) -> (sqrt(x)=w217:dbl)
        n53 = Multiply(x=w211, y=2e-05) -> (x*y=w209:dbl)
        "Sound Pressure (Pa)" <- w209
        n54 = Divide(x=w218, y=w217) -> (x/y=w210:dbl)
        n55 = Divide(x=w210, y=w209) -> (x/y=→"Sensitivity(mVeff/Pa)":dbl)
        "time record 2" <- w241
        "expected fundamental frequency [Hz]" <- w233
      }
      frame True {
        # "discard first buffer (\"0\")"
      }
    }
    n56 = flat-sequence {
      tunnel: w137 -> [w177]
      tunnel: [w178] -> w136
      tunnel: [w177] -> w86
      frame #0 {
        n57 = Tick Count (ms)() -> (millisecond timer value=w178:u32)
      }
    }
    n58 = Unbundle By Name(w137) -> ("status"=w151:bool)
    n59 = Less?(x=w125, y="Coh Faktor Thresold") -> (x < y?=w117:bool)
    n60 = case shown="True" w110 {
      tunnel: w109 -> [_ w163]
      tunnel: [0.5 ("x") w167] -> w84
      tunnel: [w158 w166] -> w85
      tunnel: [w158 w165] -> w108
      tunnel: w103 -> [_ w162]
      frame False {
        w158 = 0.5 ("x")
      }
      frame True {
        n61 = Array Subset(array=w163, index=w162, length=25) -> (w160:dbl[])
        n62 = call <vilib>:"Std Deviation and Variance.vi"("X"=w160, "Weighting (Sample)"=enum16{"Sample", "Population"}."Population") -> ("mean"=w167:dbl, "standard deviation"=w166:dbl, "variance"=w165:dbl)
      }
    }
    "standard deviation" <- w85
    n63 = Or(x=w117, y=w113) -> (x .or. y?=w116:bool)
    n64 = case shown="True" w116 {
      tunnel: w112 -> [w169 _]
      tunnel: [w169 0.0 ("THD")] -> w123
      tunnel: w121 -> [w168 w172]
      tunnel: [w168 w171] -> w120
      tunnel: w113 -> [_ w170]
      frame False {
      }
      frame True {
        n65 = case shown="False" w170 {
          tunnel: w172 -> [w175 w176]
          tunnel: [w174 w176] -> w171
          frame False {
            n66 = Increment(x=w175) -> (x+1=w174:i32)
          }
          frame True {
          }
        }
      }
    }
    "Big Sound Disturbances detected" <- w120
    n67 = Not A Number/Path/Refnum?(number/path/refnum=w82) -> (NaN/Path/Refnum?=w81:bool)
    n68 = case shown="False" w81 {
      tunnel: w84 -> [w156 _]
      tunnel: [w156 -999.0 ("mean")] -> w83
      frame False {
      }
      frame True {
      }
    }
    "mean" <- w83
    n69 = Subtract(x=w136, y=w135) -> (x-y=w93:u32)
    "loop time(ms)" <- w93
    n70 = Divide(x=w93, y=u32 1000) -> (x/y=w127:dbl)
    n71 = Add(x=w128, y=w127) -> (x+y=w89:dbl)
    n72 = Insert Into Array(array=w104, new element=w108) -> (w107:dbl[])  [unwired: 1 in]
    n73 = Insert Into Array(array=w115, new element=w125) -> (w124:dbl[])  [unwired: 1 in]
    n74 = Insert Into Array(array=w109, new element=w82) -> (w132:dbl[])  [unwired: 1 in]
    n75 = Insert Into Array(array=w105, new element=w85) -> (w96:dbl[])  [unwired: 1 in]
    n76 = Insert Into Array(array=w106, new element=w84) -> (w97:dbl[])  [unwired: 1 in]
    n77 = Insert Into Array(array=w133, new element=w89) -> (w98:dbl[])  [unwired: 1 in]
    n78 = Greater?(x=w89, y="timeout(s)") -> (0:w88:bool)
    n79 = Less?(x=w85, y="Std_Deviation_Thresold") -> (x < y?=w90:bool)
    n80 = Bundle(w98, w124) -> (w130:cluster{dbl[], dbl[]})  [unwired: 1 in]
    n81 = Bundle(w98, w132) -> (w131:cluster{dbl[], dbl[]})  [unwired: 1 in]
    n82 = Insert Into Array(array=w122, new element=w123) -> (w119:dbl[])  [unwired: 1 in]
    n83 = Bundle(w98, w96) -> (w100:cluster{dbl[], dbl[]})  [unwired: 1 in]
    n84 = Bundle(w98, w97) -> (w99:cluster{dbl[], dbl[]})  [unwired: 1 in]
    n85 = Build Array(w131, w130) -> (→"XY Graph":cluster{dbl[], dbl[]}[])
    n86 = Bundle(w98, w119) -> (→"XY Graph 2":cluster{dbl[], dbl[]})  [unwired: 1 in]
    n87 = Build Array(w99, w100) -> (→"XY Graph 3":cluster{dbl[], dbl[]}[])
    n88 = Compound Arithmetic op=OR(w151, "stop", w90, w88, w81) -> (w150:bool)
  }
  "Array" <- w16
  "Array 2" <- w3
  "Array 3" <- w2
  "Array 4" <- w1
  n89 = call <vilib>:"DAQmx Clear Task.vi"("task in"=w59, "error in"=w4) -> ("error out"=w53:errorcluster)  [unwired: 13 in]
  n90 = call-poly <vilib>:"DAQmx Write.vi"("task/channels in"=w15, "data"=w52, "error in"=w53) -> ("task out"=w51:refnum<k21>, "error out"=w50:errorcluster)  [unwired: 10 in, 1 out]
  n91 = stacked-sequence {
    tunnel: w50 -> [w253]
    tunnel: [w253] -> w49
    tunnel: w44 -> [w252]
    frame #0 {
      n92 = Wait (ms)(milliseconds to wait=w252) -> ()  [unwired: 1 out]
      n93 = global write "THD_Mess_Status.vi" "Boolean"(TRUE ("Boolean")) -> ()
    }
  }
  n94 = call <vilib>:"DAQmx Clear Task.vi"("task in"=w51, "error in"=w49) -> ("error out"=→"error out":errorcluster)  [unwired: 13 in]
